vi "CUSUM_scan_histogram_20150924.vi"() -> ()   [LabVIEW 2012]
uses:
  <vilib>/Utility/file.llb/Read From Spreadsheet File (string).vi
  <vilib>/Utility/file.llb/Read From Spreadsheet File (DBL).vi
  <vilib>/Analysis/NI_AALPro.lvlib
panel:
  out "size(s)":i32[](array[numeric])=[709, 2]
  out "Bins":dbl[](array[numeric])=[0.0, 50.0, 100.0, 150.0, 200.0, 250.0, 300.0, 350.0, 400.0, 450.0, 500.0, 550.0, 600.0, 650.0, 700.0, 750.0, 800.0, 850.0, 900.0, 950.0, 1000.0, 1050.0, 1100.0, 1150.0, 1200.0, 1250.0, 1300.0, 1350.0, 1400.0, 1450.0, 1500.0, 1550.0, 1600.0, 1650.0, 1700.0, 1750.0, 1800.0, 1850.0, 1900.0, 1950.0, 2000.0, 2050.0, 2100.0, 2150.0, 2200.0, 2250.0, 2300.0, 2350.0, 2400.0, 2450.0, 2500.0, 2550.0, 2600.0, 2650.0, 2700.0, 2750.0, 2800.0, 2850.0, 2900.0, 2950.0]
  out "level histogram 2":cluster{dbl[], dbl[]}(graph)={[0.0, 50.0, 100.0, 150.0, 200.0, 250.0, 300.0, 350.0, 400.0, 450.0, 500.0, 550.0, 600.0, 650.0, 700.0, 750.0, 800.0, 850.0, 900.0, 950.0, 1000.0, 1050.0, 1100.0, 1150.0, 1200.0, 1250.0, 1300.0, 1350.0, 1400.0, 1450.0, 1500.0, 1550.0, 1600.0, 1650.0, 1700.0, 1750.0, 1800.0, 1850.0, 1900.0, 1950.0, 2000.0, 2050.0, 2100.0, 2150.0, 2200.0, 2250.0, 2300.0, 2350.0, 2400.0, 2450.0, 2500.0, 2550.0, 2600.0, 2650.0, 2700.0, 2750.0, 2800.0, 2850.0, 2900.0, 2950.0], [0.2420675662111882, 0.0, 0.0, 0.0, 0.0, 0.0024691358024691358, 0.0, 0.0, 0.0024691358024691358, 0.0011727511965947826, 0.0024691358024691358, 0.004938750687288809, 0.007694614642743324, 0.012443819440087196, 0.01625085302825151, 0.015068413748849787, 0.018650961578816, 0.022411963620084834, 0.022281722038054834, 0.014563290150013125, 0.01687631948907472, 0.029530789836521146, 0.02262728800554096, 0.02054645698593924, 0.05519131483843338, 0.02874410635546862, 0.03054171378846674, 0.01708774938009057, 0.022621934026309416, 0.014250903106779325, 0.01999323351246907, 0.02519657870780169, 0.018748477504074733, 0.011824722459045102, 0.02938347248230296, 0.03398115844900823, 0.04379840539064302, 0.05250010646123664, 0.031092530608092937, 0.020334317018267198, 0.007966809989063132, 0.01789853994964413, 0.007181120281694738, 0.007449973130269833, 0.0049692808889797374, 0.002560338394940131, 0.00022489183940309682, 0.0025128884066004968, 0.007066785952113572, 0.0, 0.0, 0.0, 0.0, 0.0024691358024691358, 0.0, 0.0, 0.0, 0.0, 0.0, 0.0]}
  out "Array 3":dbl[](array[numeric])=[98.03736431553122, 0.0, 0.0, 0.0, 0.0, 1.0, 0.0, 0.0, 1.0, 0.474964234620887, 1.0, 2.0001940283519675, 3.116318930311046, 5.039746873235314, 6.581595476441862, 6.102707568284163, 7.553639439420479, 9.076845266134358, 9.024097425412208, 5.898132510755316, 6.834909393075262, 11.959969883791064, 9.164051642244088, 8.321315079305393, 22.35248250956552, 11.641363073964792, 12.36939408432903, 6.920538498936681, 9.161883280655314, 5.771615758245627, 8.097259572549973, 10.204614376659684, 7.593133389150267, 4.789012595913266, 11.900306355332699, 13.762369171848334, 17.738354183210426, 21.26254311680084, 12.59247489627764, 8.235398392398215, 3.2265580455705685, 7.248908679605872, 2.9083537140863687, 3.0172391177592823, 2.012558760036794, 1.036937049950753, 0.09108119495825422, 1.0177198046732012, 2.8620483106059966, 0.0, 0.0, 0.0, 0.0, 1.0, 0.0, 0.0, 0.0, 0.0, 0.0, 0.0]
  out "appended array":dbl[][](array[numeric])=[[2087.0, 0.025405017525460215], [1409.93, 0.0016283498468247178], [1971.94, 0.002677117544779621], [1432.55, 0.0038086826925730686], [2003.4, 0.020381972235255154], [1492.93, 0.0007037783236276322], [2050.7, 0.0018215438964479893], [1495.13, 0.0007037783236276322], [2012.05, 0.009563105456351945], [1732.41, 0.043703253939778655], [1965.35, 0.06242927717826291], [1520.52, 0.0046642563409047], [2060.96, 0.09819777550851434], [1503.94, 0.004802252090635608], [2016.7, 0.13191013716777522], [1660.12, 0.0037672839676537962], [2047.92, 0.04607678083515028], [1878.47, 0.11755857919576077], [2132.95, 0.0061132117130792375], [1683.32, 0.05376314409516187], [2058.8, 0.11851074986890404], [1566.97, 0.0039052797173847044], [1877.93, 0.09597604393784671], [2324.51, 0.04282008114150084], [1914.27, 0.08663373168106422], [2413.94, 0.012474815775674108], [1052.8, 1.0], [956.179, 1.0], [1638.91, 0.15711947626841244], [2420.11, 0.8428805237315876], [1509.0, 1.0], [1835.61, 0.0033733701192933964], [2231.47, 0.0014518086335808613], [1816.53, 0.06200737648138094], [2191.97, 0.0007012252720226434], [1811.18, 0.004624342388557093], [2381.62, 0.0018773094054392616], [1817.39, 0.005111115271563103], [2399.92, 0.007002040701701833], [1851.14, 0.020966976034094528], [2235.07, 0.00039826872245946255], [1827.91, 0.08563458334113418], [2355.52, 0.00041018274407149776], [1847.16, 0.012768427161926872], [2282.67, 0.0007301593245090147], [1870.95, 0.0031504077148395947], [2214.97, 6.978212658477763e-05], [1794.82, 0.0021087818253302314], [2216.53, 0.00012765023155752005], [1846.39, 0.08069026437213957], [2345.59, 0.0003676326668856577], [1817.44, 0.024369280205874293], [2371.17, 0.0006212311269132643], [1824.41, 0.014817638879196926], [2385.94, 0.002399824353281377], [1990.09, 0.000719947305984413], [1585.89, 0.00012084221920778564], [1865.83, 0.0116706351705322], [2311.3, 0.000643357167049901], [1827.78, 0.01724299327878981], [2366.37, 0.003633776591670737], [1822.67, 0.014070459523813576], [2.0, 0.00013275624081982086], [1359.57, 0.012160812059713077], [710.497, 0.0006195291238258306], [1468.34, 0.07115564307633654], [1359.72, 6.808012349734402e-05], [1726.77, 0.010816229620640532], [1859.13, 0.00010382218833344963], [2062.59, 0.0012254422229521925], [1489.94, 0.0003284865958746849], [1775.88, 0.04453291078270016], [2420.58, 0.0019913436122973127], [1908.01, 0.1268264620632022], [553.398, 0.00019402835196743047], [1419.32, 0.028874482378311035], [1067.9, 0.0013207543958484742], [1319.98, 0.0012237402198647588], [1386.9, 0.0011897001581160868], [1348.68, 0.03126920072233011], [1809.94, 0.002309618189647396], [1311.37, 0.006670150099652281], [650.96, 0.0007403713430336162], [1893.96, 0.004464354098338334], [1033.78, 0.002340254245221201], [1415.39, 0.006590155954542902], [1601.36, 0.00020424037049203208], [668.442, 0.01882415414701562], [844.813, 0.0004459248089076034], [1874.38, 0.020313406848520024], [1243.4, 0.0002723204939893761], [1500.19, 0.009672483545885152], [1908.78, 0.00046464684286937297], [781.225, 0.041836937892205335], [991.016, 0.0016032869083624519], [1368.11, 0.05483683747402318], [804.302, 0.0003267845927872513], [1580.59, 0.0023147241989096966], [1227.98, 0.0006671852102739715], [1367.09, 0.018878618245813498], [1230.17, 0.0006127211114760962], [2149.49, 0.027720524285031054], [923.501, 0.00017190231183079367], [1276.66, 0.01718342317072963], [1814.61, 0.0004918788922683106], [1405.1, 0.020568707311635064], [1376.23, 0.000473156858306541], [1966.76, 0.0028406431529266795], [2346.39, 0.00041018274407149776], [1111.97, 0.010259674611049744], [891.807, 0.007575615742166956], [899.72, 1.0], [1457.06, 1.0], [1117.79, 1.0], [921.631, 1.0], [1622.73, 1.0], [1225.74, 1.0], [1085.52, 1.0], [825.602, 1.0], [1007.3, 0.017413171379768458], [1872.61, 0.9808312772822168], [1496.45, 0.0017555513380148036], [1057.57, 1.0], [1889.63, 1.0], [1572.25, 1.0], [1234.56, 1.0], [1308.71, 1.0], [877.317, 1.0], [1907.87, 1.0], [532.884, 1.0], [560.9, 1.0], [1837.08, 1.0], [737.073, 1.0], [876.931, 1.0], [1432.36, 1.0], [993.583, 1.0], [1912.61, 1.0], [1794.02, 1.0], [1006.65, 1.0], [1036.25, 0.53125], [1896.78, 0.46875], [1241.31, 1.0], [267.724, 1.0], [1864.09, 1.0], [1112.04, 1.0], [1715.8, 1.0], [1014.02, 1.0], [1930.18, 1.0], [1560.29, 1.0], [656.028, 1.0], [682.156, 1.0], [912.345, 1.0], [1527.18, 1.0], [1627.9, 1.0], [1981.19, 0.0986159169550173], [1304.79, 0.23269896193771628], [719.808, 0.6686851211072664], [1456.22, 1.0], [1415.17, 1.0], [1870.44, 1.0], [1203.85, 1.0], [1745.38, 1.0], [1213.0, 1.0], [1933.99, 1.0], [1377.11, 1.0], [2071.24, 1.0], [1299.64, 1.0], [1606.14, 1.0], [1333.08, 1.0], [1854.4, 1.0], [1301.7, 0.17391304347826086], [1945.79, 0.8260869565217391], [1563.82, 1.0], [1910.86, 1.0], [1317.53, 1.0], [1695.63, 0.9234449760765551], [1301.8, 0.07655502392344497], [1869.95, 1.0], [1242.76, 1.0], [1788.06, 1.0], [1218.82, 1.0], [1804.39, 1.0], [1221.43, 1.0], [1810.53, 1.0], [1234.33, 1.0], [1555.4, 0.8295454545454546], [1255.86, 0.17045454545454544], [1631.74, 1.0], [1219.12, 1.0], [1684.0, 1.0], [1323.78, 0.2111111111111111], [1442.83, 0.7888888888888889], [1434.86, 1.0], [893.039, 1.0], [1474.1, 0.21739130434782608], [1657.34, 0.782608695652174], [2172.57, 1.0], [1728.16, 1.0], [2227.86, 1.0], [697.854, 1.0], [1157.3, 1.0], [851.024, 1.0], [2082.22, 1.0], [1218.51, 1.0], [1243.71, 1.0], [2094.94, 1.0], [1419.8, 0.015584415584415584], [2150.5, 0.007956600361663653], [1398.3, 0.006444188722669736], [1553.93, 0.010126582278481013], [1349.85, 0.003616636528028933], [825.641, 0.003222094361334868], [1322.58, 0.0564852868650337], [2175.33, 0.008581292125595923], [1316.6, 0.0017425612362321223], [1665.94, 0.009436133486766397], [1191.15, 0.008022357389445997], [1846.44, 0.002564524083511425], [808.1, 0.038895281933256615], [1868.78, 0.0015124116389939174], [1512.96, 0.01594607923721848], [1786.59, 0.0018083182640144665], [2325.2, 0.02857142857142857], [1783.95, 0.02314647377938517], [2290.33, 0.018411967779056387], [1778.8, 0.003090580305770179], [1461.36, 0.0010192339306263358], [1776.12, 0.00404405720861417], [1383.75, 0.022258753904323525], [2046.5, 0.003748150583593622], [1726.44, 0.00805523590333717], [2060.53, 0.003748150583593622], [1778.36, 0.0015124116389939174], [2039.58, 0.026631596251849417], [1766.09, 0.016570771001150748], [2416.11, 0.004701627486437613], [1796.06, 0.010290974847936873], [2358.84, 0.0017754397501232944], [1872.71, 0.001906953805687983], [695.836, 0.0018083182640144665], [1652.45, 0.010488245931283906], [1904.68, 0.027946736807496302], [1506.86, 0.026927502876869965], [1966.76, 0.0007562058194969587], [1978.89, 0.03524576689133651], [1397.85, 0.0012493835278645405], [1876.81, 0.003846786125267138], [940.985, 0.00496465559756699], [1864.98, 0.012230807167516029], [826.127, 0.003024823277987835], [1709.33, 0.011507479861910242], [1087.22, 0.03665954298865691], [1665.07, 0.0014795331251027453], [1506.68, 0.010685517014630939], [1800.97, 0.01818181818181818], [616.846, 0.03307578497451915], [1702.82, 0.029360512904816703], [793.399, 0.015091237876048002], [884.288, 0.016340621403912542], [810.608, 0.007266151569949039], [1895.02, 0.035771823113595266], [801.773, 0.03471971066907776], [625.159, 0.010323853361828046], [1425.1, 0.0020384678612526716], [1741.45, 0.012855498931448299], [1267.96, 0.003813907611375966], [1358.47, 0.06625020549071182], [1036.84, 0.029360512904816703], [1216.22, 0.002498767055729081], [1095.59, 0.0020055893473614993], [1612.34, 0.011704750945257275], [1690.86, 0.0020713463751438435], [645.438, 0.035147131349663], [1878.73, 0.0102580963340457], [1371.09, 0.019069538056879828], [1845.36, 0.0021042248890350158], [1213.25, 0.02975505507151077], [1477.36, 0.010685517014630939], [2093.92, 1.0], [1182.64, 1.0], [985.497, 1.0], [1612.24, 1.0], [1447.08, 1.0], [890.263, 0.01613181009242781], [722.736, 0.5019231873241863], [1935.48, 0.020265227625007175], [834.119, 0.4616797749583788], [1995.94, 1.0], [1864.17, 1.0], [1166.73, 1.0], [1955.6, 1.0], [1806.84, 1.0], [1864.15, 0.05513784461152882], [1920.31, 0.9448621553884712], [1545.9, 1.0], [1982.65, 1.0], [1836.01, 1.0], [1357.88, 1.0], [1120.61, 1.0], [1730.66, 1.0], [965.86, 0.19097395055583208], [1072.11, 0.004604280736684918], [1322.99, 0.7866268458602953], [2255.49, 0.017794922847187655], [1444.9, 1.0], [1965.5, 1.0], [644.821, 1.0], [1108.12, 1.0], [1302.96, 1.0], [1899.61, 0.0031546159893585616], [1454.0, 0.0010150499397936065], [967.774, 0.03946421285530894], [1500.54, 0.0020201484095892365], [896.694, 0.036661215472545555], [1901.57, 0.00021561518328949158], [1594.48, 0.06215024729402945], [847.541, 0.0012439337497470667], [1809.79, 0.013195649217316885], [934.503, 0.018960867502811292], [872.881, 0.0001360034233056793], [2120.85, 0.7135502532649114], [1227.66, 0.0009188523964798334], [1891.14, 0.06534466916337991], [1098.81, 0.0012704710030750042], [780.638, 0.03454818667630854], [691.653, 0.006150008458749499], [1426.0, 1.0], [553.58, 1.0], [1783.21, 0.5357142857142857], [1219.72, 0.4642857142857143], [1707.02, 0.16176470588235295], [1217.79, 0.8382352941176471], [1805.49, 1.0], [1217.83, 1.0], [1760.29, 1.0], [1215.47, 1.0], [1661.88, 1.0], [1370.49, 1.0], [1709.93, 1.0], [1216.34, 1.0], [2388.41, 1.0], [1836.91, 1.0], [2110.84, 1.0], [1895.06, 1.0], [2403.14, 1.0], [1741.31, 1.0], [1217.33, 1.0], [1784.55, 1.0], [1229.73, 1.0], [1862.39, 1.0], [806.501, 1.0], [731.362, 0.3125], [1873.14, 0.6875], [906.667, 1.0], [1082.78, 1.0], [1886.99, 1.0], [1228.77, 1.0], [1944.18, 1.0], [1885.95, 1.0], [1574.2, 1.0], [782.094, 1.0], [846.688, 1.0], [1020.4, 1.0], [965.63, 1.0], [1532.01, 1.0], [1577.86, 1.0], [2070.04, 1.0], [1292.32, 1.0], [1585.95, 1.0], [727.528, 1.0], [925.014, 1.0], [414.909, 1.0], [927.775, 1.0], [1106.07, 1.0], [2188.58, 1.0], [1868.95, 1.0], [1725.62, 1.0], [1064.71, 1.0], [813.617, 1.0], [801.414, 1.0], [797.952, 1.0], [1464.53, 0.4668574153552694], [1848.46, 0.058178350023843584], [479.276, 0.474964234620887], [717.31, 1.0], [1851.48, 1.0], [1715.99, 1.0], [1203.69, 1.0], [1200.54, 1.0], [1485.82, 1.0], [1892.21, 0.1884328358208955], [1337.15, 0.19029850746268656], [1824.55, 0.31529850746268656], [1302.31, 0.2891791044776119], [1802.99, 0.016791044776119403], [1270.27, 1.0], [1842.57, 1.0], [1282.09, 1.0], [1591.09, 1.0], [1798.15, 1.0], [1955.94, 1.0], [1282.86, 1.0], [1928.13, 1.0], [1326.64, 1.0], [1836.94, 1.0], [1235.91, 1.0], [1801.4, 1.0], [1273.72, 1.0], [1814.73, 1.0], [1302.86, 0.09285714285714286], [1825.97, 0.9071428571428571], [1463.64, 1.0], [1957.29, 1.0], [1290.55, 1.0], [1830.68, 1.0], [1345.13, 1.0], [1976.41, 1.0], [1344.34, 0.2121020154383989], [1730.56, 0.0012083245348537106], [1939.82, 0.17236808146219], [772.718, 0.0029445578470706927], [1148.21, 0.03011426292203374], [2232.36, 0.010511250322610919], [1905.87, 0.03345768517866779], [1203.01, 0.005642758264705192], [1800.68, 0.0004340583280542456], [664.521, 0.012224021022500645], [1141.53, 0.014112761314844794], [1423.25, 0.11152952769761386], [977.888, 0.06548415100537294], [1285.93, 0.0019473968231622908], [710.905, 0.05070270523920133], [1897.52, 0.04152882381924403], [1632.4, 0.01031181811782924], [1876.66, 0.1625724408155604], [1181.2, 0.0052321625489782034], [1863.87, 0.05429248492527158], [1187.18, 0.0012787123718354801], [763.809, 1.0], [1523.82, 1.0], [1034.17, 1.0], [1308.35, 1.0], [1296.01, 0.29411764705882354], [1352.97, 0.7058823529411765], [1594.5, 0.23636363636363636], [1926.88, 0.7636363636363637], [800.235, 1.0], [1014.41, 1.0], [1319.65, 1.0], [2084.98, 1.0], [1738.27, 1.0], [1066.1, 1.0], [923.378, 1.0], [2678.15, 1.0], [1368.67, 1.0], [1126.06, 1.0], [1298.0, 1.0], [2226.06, 1.0], [1084.34, 1.0], [1197.12, 1.0], [2082.17, 1.0], [1084.2, 1.0], [1825.56, 1.0], [1767.73, 1.0], [628.111, 1.0], [1847.57, 1.0], [1757.86, 1.0], [1137.1, 1.0], [1015.28, 1.0], [1879.5, 0.15833333333333333], [1720.65, 0.8416666666666667], [1251.11, 1.0], [1893.86, 1.0], [668.096, 1.0], [1779.05, 1.0], [872.978, 1.0], [1874.4, 0.004883093008559775], [1574.83, 0.02892514505658643], [1836.68, 0.009220428563221693], [1656.86, 0.00195323720342391], [2122.34, 0.15427701499396795], [1837.76, 0.0029585798816568047], [1183.61, 0.047768139254322974], [705.432, 0.002297926121675188], [639.157, 0.037772160625035904], [1874.69, 0.003159648417303384], [1176.06, 0.007066122824151203], [1401.87, 0.0642270351008215], [1375.3, 0.006204400528523008], [1807.7, 0.0053714023094157525], [1284.45, 0.1105589705290975], [1730.3, 0.010513012006663986], [1243.8, 0.004883093008559775], [1887.93, 0.006290572758085828], [1289.93, 0.04328718331705635], [1753.03, 0.0023840983512380077], [1419.85, 0.07494111564313208], [2019.86, 0.005342678232894813], [1753.86, 0.0046820244729131955], [1407.8, 0.026426150399264662], [1539.38, 0.002700063192968346], [2007.24, 0.0030734761877405643], [1163.74, 0.02260584822197966], [1946.82, 0.003504337335554662], [1965.55, 0.03211351755041075], [702.695, 0.0045096800137875565], [1701.36, 0.0055437467685413916], [1379.27, 0.0013213075199632331], [1787.09, 0.04748089848911358], [1341.8, 0.003044752111219624], [1235.84, 0.004710748549434136], [1103.74, 0.003504337335554662], [1839.3, 0.059401390245303616], [747.021, 0.006233124605043948], [743.118, 0.034124202906876545], [1797.89, 0.007238467283276842], [1793.13, 0.041132877577985866], [1426.95, 0.003705405871201241], [2125.28, 0.0066927098293789854], [1782.71, 0.016631240305624174], [2302.87, 0.018268512667317747], [846.165, 0.0028149594990521053], [1397.34, 0.004251163325099098], [756.643, 1.0], [1183.51, 1.0], [786.257, 1.0], [781.436, 1.0], [690.436, 1.0], [1085.61, 1.0], [1480.42, 1.0], [1772.17, 1.0], [1768.87, 1.0], [1128.08, 1.0], [1780.1, 1.0], [1585.3, 1.0], [1270.53, 1.0], [906.421, 1.0], [1911.6, 1.0], [1357.53, 1.0], [1840.69, 1.0], [836.077, 1.0], [1310.64, 1.0], [1881.75, 1.0], [2187.62, 1.0], [1534.2, 1.0], [1152.6, 1.0], [965.228, 1.0], [907.996, 1.0], [1049.23, 0.2545454545454545], [1711.8, 0.7454545454545455], [2030.86, 1.0], [1853.24, 1.0], [1064.62, 0.020169851380042462], [2026.48, 0.9798301486199575], [1169.14, 1.0], [2425.73, 1.0], [2266.82, 1.0], [893.285, 1.0], [1299.6, 1.0], [1615.69, 1.0], [1955.45, 1.0], [1084.31, 1.0], [1546.11, 1.0], [1529.82, 1.0], [1816.24, 1.0], [2148.28, 1.0], [1410.36, 1.0], [1552.85, 1.0], [1781.22, 1.0], [1780.3, 1.0], [1697.19, 1.0], [1190.53, 1.0], [1069.78, 0.8939393939393939], [1108.17, 0.10606060606060606], [1851.27, 1.0], [1342.98, 1.0], [850.381, 1.0], [1854.66, 1.0], [1398.03, 1.0], [1100.29, 1.0], [2016.17, 1.0], [1625.97, 0.41379310344827586], [1941.51, 0.5862068965517241], [701.989, 1.0], [1930.6, 1.0], [1708.51, 1.0], [942.204, 1.0], [1067.87, 1.0], [709.937, 1.0], [1600.57, 1.0], [1412.42, 1.0], [648.139, 1.0], [1877.51, 1.0], [885.259, 1.0], [954.4, 0.03443043884220355], [997.229, 0.39017273576097106], [1723.12, 0.017857142857142856], [1855.66, 0.042600373482726425], [974.682, 0.035130718954248366], [1400.0, 0.013071895424836602], [753.804, 0.008286647992530346], [1554.74, 0.031162464985994398], [986.868, 0.14087301587301587], [1524.19, 0.01984126984126984], [1155.7, 0.22934173669467786], [0.0, 0.03723155929038282], [0.0, 0.07675438596491228], [0.0, 0.9232456140350878], [0.0, 1.0], [0.0, 1.0], [0.0, 1.0], [0.0, 1.0], [0.0, 1.0], [0.0, 1.0], [0.0, 1.0], [0.0, 1.0], [0.0, 1.0], [0.0, 1.0], [0.0, 1.0], [0.0, 1.0], [0.0, 1.0], [0.0, 1.0], [0.0, 1.0], [0.0, 1.0], [0.0, 1.0], [0.0, 1.0], [0.0, 1.0], [0.0, 1.0], [0.0, 1.0], [0.0, 1.0], [0.0, 1.0], [0.0, 1.0], [0.0, 1.0], [0.0, 1.0], [0.0, 1.0], [0.0, 1.0], [0.0, 1.0], [0.0, 1.0], [0.0, 1.0], [0.0, 1.0], [0.0, 1.0], [0.0, 1.0], [0.0, 1.0], [0.0, 1.0], [0.0, 1.0], [0.0, 0.03875], [0.0, 0.87125], [0.0, 0.09], [0.0, 1.0], [0.0, 1.0], [0.0, 1.0], [0.0, 1.0], [0.0, 1.0], [0.0, 0.2927170868347339], [0.0, 0.7072829131652661], [0.0, 1.0], [0.0, 1.0], [0.0, 1.0], [0.0, 1.0], [0.0, 1.0], [0.0, 1.0], [0.0, 1.0], [0.0, 1.0], [0.0, 1.0], [0.0, 1.0], [0.0, 1.0], [0.0, 1.0], [0.0, 1.0], [0.0, 0.46153846153846156], [0.0, 0.5384615384615384], [0.0, 1.0], [0.0, 1.0], [0.0, 1.0], [0.0, 1.0], [0.0, 1.0], [0.0, 1.0], [0.0, 1.0], [0.0, 1.0], [0.0, 1.0], [0.0, 1.0], [0.0, 1.0], [0.0, 1.0], [0.0, 1.0], [0.0, 1.0], [0.0, 1.0], [0.0, 1.0], [0.0, 1.0], [0.0, 1.0], [0.0, 1.0], [0.0, 1.0], [0.0, 1.0], [0.0, 1.0], [0.0, 1.0], [0.0, 1.0], [0.0, 1.0], [0.0, 1.0], [0.0, 1.0], [0.0, 1.0], [0.0, 1.0], [0.0, 1.0], [0.0, 1.0], [0.0, 1.0], [0.0, 1.0], [0.0, 1.0], [0.0, 1.0], [0.0, 1.0], [0.0, 1.0], [0.0, 1.0], [0.0, 1.0]]
  out "Array 2":dbl[](array[numeric])=[0.025405017525460215, 0.0016283498468247178, 0.002677117544779621, 0.0038086826925730686, 0.020381972235255154, 0.0007037783236276322, 0.0018215438964479893, 0.0007037783236276322, 0.009563105456351945, 0.043703253939778655, 0.06242927717826291, 0.0046642563409047, 0.09819777550851434, 0.004802252090635608, 0.13191013716777522, 0.0037672839676537962, 0.04607678083515028, 0.11755857919576077, 0.0061132117130792375, 0.05376314409516187, 0.11851074986890404, 0.0039052797173847044, 0.09597604393784671, 0.04282008114150084, 0.08663373168106422, 0.012474815775674108, 1.0, 1.0, 0.15711947626841244, 0.8428805237315876, 1.0, 0.0033733701192933964, 0.0014518086335808613, 0.06200737648138094, 0.0007012252720226434, 0.004624342388557093, 0.0018773094054392616, 0.005111115271563103, 0.007002040701701833, 0.020966976034094528, 0.00039826872245946255, 0.08563458334113418, 0.00041018274407149776, 0.012768427161926872, 0.0007301593245090147, 0.0031504077148395947, 6.978212658477763e-05, 0.0021087818253302314, 0.00012765023155752005, 0.08069026437213957, 0.0003676326668856577, 0.024369280205874293, 0.0006212311269132643, 0.014817638879196926, 0.002399824353281377, 0.000719947305984413, 0.00012084221920778564, 0.0116706351705322, 0.000643357167049901, 0.01724299327878981, 0.003633776591670737, 0.014070459523813576, 0.00013275624081982086, 0.012160812059713077, 0.0006195291238258306, 0.07115564307633654, 6.808012349734402e-05, 0.010816229620640532, 0.00010382218833344963, 0.0012254422229521925, 0.0003284865958746849, 0.04453291078270016, 0.0019913436122973127, 0.1268264620632022, 0.00019402835196743047, 0.028874482378311035, 0.0013207543958484742, 0.0012237402198647588, 0.0011897001581160868, 0.03126920072233011, 0.002309618189647396, 0.006670150099652281, 0.0007403713430336162, 0.004464354098338334, 0.002340254245221201, 0.006590155954542902, 0.00020424037049203208, 0.01882415414701562, 0.0004459248089076034, 0.020313406848520024, 0.0002723204939893761, 0.009672483545885152, 0.00046464684286937297, 0.041836937892205335, 0.0016032869083624519, 0.05483683747402318, 0.0003267845927872513, 0.0023147241989096966, 0.0006671852102739715, 0.018878618245813498, 0.0006127211114760962, 0.027720524285031054, 0.00017190231183079367, 0.01718342317072963, 0.0004918788922683106, 0.020568707311635064, 0.000473156858306541, 0.0028406431529266795, 0.00041018274407149776, 0.010259674611049744, 0.007575615742166956, 1.0, 1.0, 1.0, 1.0, 1.0, 1.0, 1.0, 1.0, 0.017413171379768458, 0.9808312772822168, 0.0017555513380148036, 1.0, 1.0, 1.0, 1.0, 1.0, 1.0, 1.0, 1.0, 1.0, 1.0, 1.0, 1.0, 1.0, 1.0, 1.0, 1.0, 1.0, 0.53125, 0.46875, 1.0, 1.0, 1.0, 1.0, 1.0, 1.0, 1.0, 1.0, 1.0, 1.0, 1.0, 1.0, 1.0, 0.0986159169550173, 0.23269896193771628, 0.6686851211072664, 1.0, 1.0, 1.0, 1.0, 1.0, 1.0, 1.0, 1.0, 1.0, 1.0, 1.0, 1.0, 1.0, 0.17391304347826086, 0.8260869565217391, 1.0, 1.0, 1.0, 0.9234449760765551, 0.07655502392344497, 1.0, 1.0, 1.0, 1.0, 1.0, 1.0, 1.0, 1.0, 0.8295454545454546, 0.17045454545454544, 1.0, 1.0, 1.0, 0.2111111111111111, 0.7888888888888889, 1.0, 1.0, 0.21739130434782608, 0.782608695652174, 1.0, 1.0, 1.0, 1.0, 1.0, 1.0, 1.0, 1.0, 1.0, 1.0, 0.015584415584415584, 0.007956600361663653, 0.006444188722669736, 0.010126582278481013, 0.003616636528028933, 0.003222094361334868, 0.0564852868650337, 0.008581292125595923, 0.0017425612362321223, 0.009436133486766397, 0.008022357389445997, 0.002564524083511425, 0.038895281933256615, 0.0015124116389939174, 0.01594607923721848, 0.0018083182640144665, 0.02857142857142857, 0.02314647377938517, 0.018411967779056387, 0.003090580305770179, 0.0010192339306263358, 0.00404405720861417, 0.022258753904323525, 0.003748150583593622, 0.00805523590333717, 0.003748150583593622, 0.0015124116389939174, 0.026631596251849417, 0.016570771001150748, 0.004701627486437613, 0.010290974847936873, 0.0017754397501232944, 0.001906953805687983, 0.0018083182640144665, 0.010488245931283906, 0.027946736807496302, 0.026927502876869965, 0.0007562058194969587, 0.03524576689133651, 0.0012493835278645405, 0.003846786125267138, 0.00496465559756699, 0.012230807167516029, 0.003024823277987835, 0.011507479861910242, 0.03665954298865691, 0.0014795331251027453, 0.010685517014630939, 0.01818181818181818, 0.03307578497451915, 0.029360512904816703, 0.015091237876048002, 0.016340621403912542, 0.007266151569949039, 0.035771823113595266, 0.03471971066907776, 0.010323853361828046, 0.0020384678612526716, 0.012855498931448299, 0.003813907611375966, 0.06625020549071182, 0.029360512904816703, 0.002498767055729081, 0.0020055893473614993, 0.011704750945257275, 0.0020713463751438435, 0.035147131349663, 0.0102580963340457, 0.019069538056879828, 0.0021042248890350158, 0.02975505507151077, 0.010685517014630939, 1.0, 1.0, 1.0, 1.0, 1.0, 0.01613181009242781, 0.5019231873241863, 0.020265227625007175, 0.4616797749583788, 1.0, 1.0, 1.0, 1.0, 1.0, 0.05513784461152882, 0.9448621553884712, 1.0, 1.0, 1.0, 1.0, 1.0, 1.0, 0.19097395055583208, 0.004604280736684918, 0.7866268458602953, 0.017794922847187655, 1.0, 1.0, 1.0, 1.0, 1.0, 0.0031546159893585616, 0.0010150499397936065, 0.03946421285530894, 0.0020201484095892365, 0.036661215472545555, 0.00021561518328949158, 0.06215024729402945, 0.0012439337497470667, 0.013195649217316885, 0.018960867502811292, 0.0001360034233056793, 0.7135502532649114, 0.0009188523964798334, 0.06534466916337991, 0.0012704710030750042, 0.03454818667630854, 0.006150008458749499, 1.0, 1.0, 0.5357142857142857, 0.4642857142857143, 0.16176470588235295, 0.8382352941176471, 1.0, 1.0, 1.0, 1.0, 1.0, 1.0, 1.0, 1.0, 1.0, 1.0, 1.0, 1.0, 1.0, 1.0, 1.0, 1.0, 1.0, 1.0, 1.0, 0.3125, 0.6875, 1.0, 1.0, 1.0, 1.0, 1.0, 1.0, 1.0, 1.0, 1.0, 1.0, 1.0, 1.0, 1.0, 1.0, 1.0, 1.0, 1.0, 1.0, 1.0, 1.0, 1.0, 1.0, 1.0, 1.0, 1.0, 1.0, 1.0, 1.0, 0.4668574153552694, 0.058178350023843584, 0.474964234620887, 1.0, 1.0, 1.0, 1.0, 1.0, 1.0, 0.1884328358208955, 0.19029850746268656, 0.31529850746268656, 0.2891791044776119, 0.016791044776119403, 1.0, 1.0, 1.0, 1.0, 1.0, 1.0, 1.0, 1.0, 1.0, 1.0, 1.0, 1.0, 1.0, 1.0, 0.09285714285714286, 0.9071428571428571, 1.0, 1.0, 1.0, 1.0, 1.0, 1.0, 0.2121020154383989, 0.0012083245348537106, 0.17236808146219, 0.0029445578470706927, 0.03011426292203374, 0.010511250322610919, 0.03345768517866779, 0.005642758264705192, 0.0004340583280542456, 0.012224021022500645, 0.014112761314844794, 0.11152952769761386, 0.06548415100537294, 0.0019473968231622908, 0.05070270523920133, 0.04152882381924403, 0.01031181811782924, 0.1625724408155604, 0.0052321625489782034, 0.05429248492527158, 0.0012787123718354801, 1.0, 1.0, 1.0, 1.0, 0.29411764705882354, 0.7058823529411765, 0.23636363636363636, 0.7636363636363637, 1.0, 1.0, 1.0, 1.0, 1.0, 1.0, 1.0, 1.0, 1.0, 1.0, 1.0, 1.0, 1.0, 1.0, 1.0, 1.0, 1.0, 1.0, 1.0, 1.0, 1.0, 1.0, 1.0, 0.15833333333333333, 0.8416666666666667, 1.0, 1.0, 1.0, 1.0, 1.0, 0.004883093008559775, 0.02892514505658643, 0.009220428563221693, 0.00195323720342391, 0.15427701499396795, 0.0029585798816568047, 0.047768139254322974, 0.002297926121675188, 0.037772160625035904, 0.003159648417303384, 0.007066122824151203, 0.0642270351008215, 0.006204400528523008, 0.0053714023094157525, 0.1105589705290975, 0.010513012006663986, 0.004883093008559775, 0.006290572758085828, 0.04328718331705635, 0.0023840983512380077, 0.07494111564313208, 0.005342678232894813, 0.0046820244729131955, 0.026426150399264662, 0.002700063192968346, 0.0030734761877405643, 0.02260584822197966, 0.003504337335554662, 0.03211351755041075, 0.0045096800137875565, 0.0055437467685413916, 0.0013213075199632331, 0.04748089848911358, 0.003044752111219624, 0.004710748549434136, 0.003504337335554662, 0.059401390245303616, 0.006233124605043948, 0.034124202906876545, 0.007238467283276842, 0.041132877577985866, 0.003705405871201241, 0.0066927098293789854, 0.016631240305624174, 0.018268512667317747, 0.0028149594990521053, 0.004251163325099098, 1.0, 1.0, 1.0, 1.0, 1.0, 1.0, 1.0, 1.0, 1.0, 1.0, 1.0, 1.0, 1.0, 1.0, 1.0, 1.0, 1.0, 1.0, 1.0, 1.0, 1.0, 1.0, 1.0, 1.0, 1.0, 0.2545454545454545, 0.7454545454545455, 1.0, 1.0, 0.020169851380042462, 0.9798301486199575, 1.0, 1.0, 1.0, 1.0, 1.0, 1.0, 1.0, 1.0, 1.0, 1.0, 1.0, 1.0, 1.0, 1.0, 1.0, 1.0, 1.0, 1.0, 0.8939393939393939, 0.10606060606060606, 1.0, 1.0, 1.0, 1.0, 1.0, 1.0, 1.0, 0.41379310344827586, 0.5862068965517241, 1.0, 1.0, 1.0, 1.0, 1.0, 1.0, 1.0, 1.0, 1.0, 1.0, 1.0, 0.03443043884220355, 0.39017273576097106, 0.017857142857142856, 0.042600373482726425, 0.035130718954248366, 0.013071895424836602, 0.008286647992530346, 0.031162464985994398, 0.14087301587301587, 0.01984126984126984, 0.22934173669467786, 0.03723155929038282, 0.07675438596491228, 0.9232456140350878, 1.0, 1.0, 1.0, 1.0, 1.0, 1.0, 1.0, 1.0, 1.0, 1.0, 1.0, 1.0, 1.0, 1.0, 1.0, 1.0, 1.0, 1.0, 1.0, 1.0, 1.0, 1.0, 1.0, 1.0, 1.0, 1.0, 1.0, 1.0, 1.0, 1.0, 1.0, 1.0, 1.0, 1.0, 1.0, 1.0, 1.0, 0.03875, 0.87125, 0.09, 1.0, 1.0, 1.0, 1.0, 1.0, 0.2927170868347339, 0.7072829131652661, 1.0, 1.0, 1.0, 1.0, 1.0, 1.0, 1.0, 1.0, 1.0, 1.0, 1.0, 1.0, 1.0, 0.46153846153846156, 0.5384615384615384, 1.0, 1.0, 1.0, 1.0, 1.0, 1.0, 1.0, 1.0, 1.0, 1.0, 1.0, 1.0, 1.0, 1.0, 1.0, 1.0, 1.0, 1.0, 1.0, 1.0, 1.0, 1.0, 1.0, 1.0, 1.0, 1.0, 1.0, 1.0, 1.0, 1.0, 1.0, 1.0, 1.0, 1.0, 1.0, 1.0, 1.0, 1.0, 1.0]
  out "Array":dbl[](array[numeric])=[2087.0, 1409.93, 1971.94, 1432.55, 2003.4, 1492.93, 2050.7, 1495.13, 2012.05, 1732.41, 1965.35, 1520.52, 2060.96, 1503.94, 2016.7, 1660.12, 2047.92, 1878.47, 2132.95, 1683.32, 2058.8, 1566.97, 1877.93, 2324.51, 1914.27, 2413.94, 1052.8, 956.179, 1638.91, 2420.11, 1509.0, 1835.61, 2231.47, 1816.53, 2191.97, 1811.18, 2381.62, 1817.39, 2399.92, 1851.14, 2235.07, 1827.91, 2355.52, 1847.16, 2282.67, 1870.95, 2214.97, 1794.82, 2216.53, 1846.39, 2345.59, 1817.44, 2371.17, 1824.41, 2385.94, 1990.09, 1585.89, 1865.83, 2311.3, 1827.78, 2366.37, 1822.67, 2.0, 1359.57, 710.497, 1468.34, 1359.72, 1726.77, 1859.13, 2062.59, 1489.94, 1775.88, 2420.58, 1908.01, 553.398, 1419.32, 1067.9, 1319.98, 1386.9, 1348.68, 1809.94, 1311.37, 650.96, 1893.96, 1033.78, 1415.39, 1601.36, 668.442, 844.813, 1874.38, 1243.4, 1500.19, 1908.78, 781.225, 991.016, 1368.11, 804.302, 1580.59, 1227.98, 1367.09, 1230.17, 2149.49, 923.501, 1276.66, 1814.61, 1405.1, 1376.23, 1966.76, 2346.39, 1111.97, 891.807, 899.72, 1457.06, 1117.79, 921.631, 1622.73, 1225.74, 1085.52, 825.602, 1007.3, 1872.61, 1496.45, 1057.57, 1889.63, 1572.25, 1234.56, 1308.71, 877.317, 1907.87, 532.884, 560.9, 1837.08, 737.073, 876.931, 1432.36, 993.583, 1912.61, 1794.02, 1006.65, 1036.25, 1896.78, 1241.31, 267.724, 1864.09, 1112.04, 1715.8, 1014.02, 1930.18, 1560.29, 656.028, 682.156, 912.345, 1527.18, 1627.9, 1981.19, 1304.79, 719.808, 1456.22, 1415.17, 1870.44, 1203.85, 1745.38, 1213.0, 1933.99, 1377.11, 2071.24, 1299.64, 1606.14, 1333.08, 1854.4, 1301.7, 1945.79, 1563.82, 1910.86, 1317.53, 1695.63, 1301.8, 1869.95, 1242.76, 1788.06, 1218.82, 1804.39, 1221.43, 1810.53, 1234.33, 1555.4, 1255.86, 1631.74, 1219.12, 1684.0, 1323.78, 1442.83, 1434.86, 893.039, 1474.1, 1657.34, 2172.57, 1728.16, 2227.86, 697.854, 1157.3, 851.024, 2082.22, 1218.51, 1243.71, 2094.94, 1419.8, 2150.5, 1398.3, 1553.93, 1349.85, 825.641, 1322.58, 2175.33, 1316.6, 1665.94, 1191.15, 1846.44, 808.1, 1868.78, 1512.96, 1786.59, 2325.2, 1783.95, 2290.33, 1778.8, 1461.36, 1776.12, 1383.75, 2046.5, 1726.44, 2060.53, 1778.36, 2039.58, 1766.09, 2416.11, 1796.06, 2358.84, 1872.71, 695.836, 1652.45, 1904.68, 1506.86, 1966.76, 1978.89, 1397.85, 1876.81, 940.985, 1864.98, 826.127, 1709.33, 1087.22, 1665.07, 1506.68, 1800.97, 616.846, 1702.82, 793.399, 884.288, 810.608, 1895.02, 801.773, 625.159, 1425.1, 1741.45, 1267.96, 1358.47, 1036.84, 1216.22, 1095.59, 1612.34, 1690.86, 645.438, 1878.73, 1371.09, 1845.36, 1213.25, 1477.36, 2093.92, 1182.64, 985.497, 1612.24, 1447.08, 890.263, 722.736, 1935.48, 834.119, 1995.94, 1864.17, 1166.73, 1955.6, 1806.84, 1864.15, 1920.31, 1545.9, 1982.65, 1836.01, 1357.88, 1120.61, 1730.66, 965.86, 1072.11, 1322.99, 2255.49, 1444.9, 1965.5, 644.821, 1108.12, 1302.96, 1899.61, 1454.0, 967.774, 1500.54, 896.694, 1901.57, 1594.48, 847.541, 1809.79, 934.503, 872.881, 2120.85, 1227.66, 1891.14, 1098.81, 780.638, 691.653, 1426.0, 553.58, 1783.21, 1219.72, 1707.02, 1217.79, 1805.49, 1217.83, 1760.29, 1215.47, 1661.88, 1370.49, 1709.93, 1216.34, 2388.41, 1836.91, 2110.84, 1895.06, 2403.14, 1741.31, 1217.33, 1784.55, 1229.73, 1862.39, 806.501, 731.362, 1873.14, 906.667, 1082.78, 1886.99, 1228.77, 1944.18, 1885.95, 1574.2, 782.094, 846.688, 1020.4, 965.63, 1532.01, 1577.86, 2070.04, 1292.32, 1585.95, 727.528, 925.014, 414.909, 927.775, 1106.07, 2188.58, 1868.95, 1725.62, 1064.71, 813.617, 801.414, 797.952, 1464.53, 1848.46, 479.276, 717.31, 1851.48, 1715.99, 1203.69, 1200.54, 1485.82, 1892.21, 1337.15, 1824.55, 1302.31, 1802.99, 1270.27, 1842.57, 1282.09, 1591.09, 1798.15, 1955.94, 1282.86, 1928.13, 1326.64, 1836.94, 1235.91, 1801.4, 1273.72, 1814.73, 1302.86, 1825.97, 1463.64, 1957.29, 1290.55, 1830.68, 1345.13, 1976.41, 1344.34, 1730.56, 1939.82, 772.718, 1148.21, 2232.36, 1905.87, 1203.01, 1800.68, 664.521, 1141.53, 1423.25, 977.888, 1285.93, 710.905, 1897.52, 1632.4, 1876.66, 1181.2, 1863.87, 1187.18, 763.809, 1523.82, 1034.17, 1308.35, 1296.01, 1352.97, 1594.5, 1926.88, 800.235, 1014.41, 1319.65, 2084.98, 1738.27, 1066.1, 923.378, 2678.15, 1368.67, 1126.06, 1298.0, 2226.06, 1084.34, 1197.12, 2082.17, 1084.2, 1825.56, 1767.73, 628.111, 1847.57, 1757.86, 1137.1, 1015.28, 1879.5, 1720.65, 1251.11, 1893.86, 668.096, 1779.05, 872.978, 1874.4, 1574.83, 1836.68, 1656.86, 2122.34, 1837.76, 1183.61, 705.432, 639.157, 1874.69, 1176.06, 1401.87, 1375.3, 1807.7, 1284.45, 1730.3, 1243.8, 1887.93, 1289.93, 1753.03, 1419.85, 2019.86, 1753.86, 1407.8, 1539.38, 2007.24, 1163.74, 1946.82, 1965.55, 702.695, 1701.36, 1379.27, 1787.09, 1341.8, 1235.84, 1103.74, 1839.3, 747.021, 743.118, 1797.89, 1793.13, 1426.95, 2125.28, 1782.71, 2302.87, 846.165, 1397.34, 756.643, 1183.51, 786.257, 781.436, 690.436, 1085.61, 1480.42, 1772.17, 1768.87, 1128.08, 1780.1, 1585.3, 1270.53, 906.421, 1911.6, 1357.53, 1840.69, 836.077, 1310.64, 1881.75, 2187.62, 1534.2, 1152.6, 965.228, 907.996, 1049.23, 1711.8, 2030.86, 1853.24, 1064.62, 2026.48, 1169.14, 2425.73, 2266.82, 893.285, 1299.6, 1615.69, 1955.45, 1084.31, 1546.11, 1529.82, 1816.24, 2148.28, 1410.36, 1552.85, 1781.22, 1780.3, 1697.19, 1190.53, 1069.78, 1108.17, 1851.27, 1342.98, 850.381, 1854.66, 1398.03, 1100.29, 2016.17, 1625.97, 1941.51, 701.989, 1930.6, 1708.51, 942.204, 1067.87, 709.937, 1600.57, 1412.42, 648.139, 1877.51, 885.259, 954.4, 997.229, 1723.12, 1855.66, 974.682, 1400.0, 753.804, 1554.74, 986.868, 1524.19, 1155.7]
  out "bin size":dbl=50.0
  in  "Min blockage (pA) 2":dbl format="%0.2f"
  in  "Max blockage (pA) 2":dbl=3000.0 format="%0.2f"
  in  "CUSUM levels histogram 2":bool=TRUE
  out "Scatter density":i32[][](graph)
  in  "Log t":bool=TRUE
  in  "Min I (pA)":dbl format="%_3g"
  in  "Max I (pA)":dbl=1.0 format="%_3g"
  in  "Current bins":i16=100
  in  "t Min (us)":dbl=1.0 format="%_3g"
  in  "t Max (us)":dbl=2000000.0 format="%_3g"
  in  "t Bins":i16=100
  out "Blockage vs Event time":cluster{"all rows":dbl[], "all rows":dbl[]}(graph)
  in  "Scatter plot":bool=TRUE
  in  "stop 2":bool
  in  "stop":bool
  in  "Dwell time min bin":dbl format="%0.2f"
  in  "Dwell time max bin":dbl=500.0 format="%0.2f"
  in  "Max block min (pA)":dbl format="%0.2f"
  in  "Max block max (pA)":dbl=1.0 format="%0.2f"
  in  "#bins (max block)":i32=50
  out "Max blockage (pA)":T1(graph)={"X Values"=[0.01, 0.03, 0.05, 0.07, 0.09, 0.11, 0.13, 0.15000000000000002, 0.16999999999999998, 0.19, 0.21000000000000002, 0.22999999999999998, 0.25, 0.27, 0.29000000000000004, 0.31, 0.33, 0.35, 0.37, 0.39, 0.41000000000000003, 0.43, 0.45, 0.47, 0.49, 0.51, 0.53, 0.55, 0.5700000000000001, 0.59, 0.61, 0.63, 0.65, 0.67, 0.6900000000000001, 0.71, 0.73, 0.75, 0.77, 0.79, 0.81, 0.8300000000000001, 0.85, 0.87, 0.89, 0.91, 0.93, 0.95, 0.97, 0.99], "Histogram: h(x)"=[0.0, 0.0, 0.0, 0.0, 0.0, 0.0, 0.0, 0.0024937655860349127, 0.0024937655860349127, 0.007481296758104738, 0.0024937655860349127, 0.02493765586034913, 0.03740648379052369, 0.032418952618453865, 0.04239401496259352, 0.032418952618453865, 0.03740648379052369, 0.032418952618453865, 0.022443890274314215, 0.057356608478802994, 0.02743142144638404, 0.0399002493765586, 0.022443890274314215, 0.029925187032418952, 0.04738154613466334, 0.03740648379052369, 0.032418952618453865, 0.02743142144638404, 0.032418952618453865, 0.014962593516209476, 0.029925187032418952, 0.032418952618453865, 0.03740648379052369, 0.08728179551122195, 0.05236907730673317, 0.02493765586034913, 0.007481296758104738, 0.02493765586034913, 0.012468827930174564, 0.007481296758104738, 0.012468827930174564, 0.0024937655860349127, 0.0024937655860349127, 0.017456359102244388, 0.0, 0.0, 0.0, 0.0, 0.0024937655860349127, 0.0]}
  out "Dwell time (us)":cluster{"Axis":dbl[], dbl[]}[](graph)=[{"Axis"=[5.0, 15.0, 25.0, 35.0, 45.0, 55.0, 65.0, 75.0, 85.0, 95.0, 105.0, 115.0, 125.0, 135.0, 145.0, 155.0, 165.0, 175.0, 185.0, 195.0, 205.0, 215.0, 225.0, 235.0, 245.0, 255.0, 265.0, 275.0, 285.0, 295.0, 305.0, 315.0, 325.0, 335.0, 345.0, 355.0, 365.0, 375.0, 385.0, 395.0, 405.0, 415.0, 425.0, 435.0, 445.0, 455.0, 465.0, 475.0, 485.0, 495.0], [47.0, 203.0, 25.0, 12.0, 11.0, 7.0, 6.0, 9.0, 7.0, 9.0, 2.0, 6.0, 5.0, 9.0, 0.0, 1.0, 4.0, 3.0, 3.0, 1.0, 0.0, 1.0, 0.0, 0.0, 1.0, 0.0, 0.0, 1.0, 1.0, 0.0, 0.0, 0.0, 0.0, 0.0, 1.0, 0.0, 0.0, 0.0, 0.0, 0.0, 0.0, 1.0, 0.0, 0.0, 0.0, 0.0, 1.0, 0.0, 1.0, 0.0]}, {"Axis"=[5.0, 15.0, 25.0, 35.0, 45.0, 55.0, 65.0, 75.0, 85.0, 95.0, 105.0, 115.0, 125.0, 135.0, 145.0, 155.0, 165.0, 175.0, 185.0, 195.0, 205.0, 215.0, 225.0, 235.0, 245.0, 255.0, 265.0, 275.0, 285.0, 295.0, 305.0, 315.0, 325.0, 335.0, 345.0, 355.0, 365.0, 375.0, 385.0, 395.0, 405.0, 415.0, 425.0, 435.0, 445.0, 455.0, 465.0, 475.0, 485.0, 495.0], [0.12433862433862433, 0.5370370370370371, 0.06613756613756613, 0.031746031746031744, 0.0291005291005291, 0.018518518518518517, 0.015873015873015872, 0.023809523809523808, 0.018518518518518517, 0.023809523809523808, 0.005291005291005291, 0.015873015873015872, 0.013227513227513227, 0.023809523809523808, 0.0, 0.0026455026455026454, 0.010582010582010581, 0.007936507936507936, 0.007936507936507936, 0.0026455026455026454, 0.0, 0.0026455026455026454, 0.0, 0.0, 0.0026455026455026454, 0.0, 0.0, 0.0026455026455026454, 0.0026455026455026454, 0.0, 0.0, 0.0, 0.0, 0.0, 0.0026455026455026454, 0.0, 0.0, 0.0, 0.0, 0.0, 0.0, 0.0026455026455026454, 0.0, 0.0, 0.0, 0.0, 0.0026455026455026454, 0.0, 0.0026455026455026454, 0.0]}]
  out "min dwell time":dbl=4.0
  out "max dwell time":dbl=1180000.0
  in  "#bins (dwell)":i32=50
  in  "Max blockage histogram":bool=TRUE
  in  "Dwell time histogram":bool=TRUE
  out "Events analysed":i32
  out "sum (dummy check)":dbl=0.9963822472223787
  out "event length":i32=216
  out "Histogram":i32[](array[numeric])=[0, 0, 0, 0, 0, 0, 0, 0, 0, 0, 0, 1, 0, 0, 0, 0, 0, 0, 0, 0, 0, 0, 0, 0, 0, 0, 0, 0, 0, 0, 0, 0, 0, 0, 0, 0, 0, 0, 0, 0, 0, 0, 0, 0, 0, 0, 0, 0, 0, 0]
  out "Levels histogram":cluster{"Axis":dbl[], dbl[]}(graph)={"Axis"=[-3465.0, -3395.0, -3325.0, -3255.0, -3185.0, -3115.0, -3045.0, -2975.0, -2905.0, -2835.0, -2765.0, -2695.0, -2625.0, -2555.0, -2485.0, -2415.0, -2345.0, -2275.0, -2205.0, -2135.0, -2065.0, -1995.0, -1925.0, -1855.0, -1785.0, -1715.0, -1645.0, -1575.0, -1505.0, -1435.0, -1365.0, -1295.0, -1225.0, -1155.0, -1085.0, -1015.0, -945.0, -875.0, -805.0, -735.0, -665.0, -595.0, -525.0, -455.0, -385.0, -315.0, -245.0, -175.0, -105.0, -35.0], [0.0004949710534058188, 0.0005575107571682827, 0.0001833475976425106, 0.00031649062619960714, 0.0009038635940800331, 0.0009151745206729308, 0.0008976400417446829, 0.0016365757773167046, 0.0033132967394204757, 0.005761032897407708, 0.025661984455272346, 0.3536324808135091, 0.4010886480266952, 0.04444740968906965, 0.00610171878792866, 0.001842720890428927, 0.0011289414947405505, 0.0008389566023915335, 0.0011172240577151799, 0.0005197184732067511, 0.0006034201729588347, 0.0004933665394832644, 0.00032185808538917843, 0.0006615560073560593, 0.0005686703564385492, 0.0009888549020411514, 0.0007824467779992721, 0.0016983786202295686, 0.0020475788830917017, 0.0015802329978052941, 0.005471286054086217, 0.006872608057804315, 0.0025711244937169754, 0.006312800625638749, 0.00696186076810715, 0.006686656172749102, 0.011719105900513196, 0.03457162380260294, 0.025076556913255776, 0.005739451255138987, 0.006988723622568358, 0.0054167527145173285, 0.003024455202881837, 0.004714153538480746, 0.0017621018281088823, 0.001344500548197642, 1.1613322803920659e-05, 0.0, 1.1446624390467251e-05, 1.935553800653443e-05]}
  out "Cumulative histogram":i32[](array[numeric])
  in  "# bins":i32=60
  in  "Min current (pA)":dbl=-3500.0 format="%0.2f"
  in  "Max current (pA)":dbl format="%0.2f"
  in  "CUSUM levels histogram":bool
  out "Event details":dbl[](array[numeric])=[5.231562, 144932.0, 2413.94, 26.0] caption="Time (s)\n      Length (us)\nMax block (pA)   \n           # levels"
  out "CUSUM event":path=path "D:/DATA/2015/Sep2015/sep22/1705_10111_36MLiClpH8_3uLlane1dsDNA_150mV/events/event_00000.csv"
  out "CUSUM event":cluster{"Y":dbl[], "Y":dbl[]}[](graph)
  in  "Event Index":i32
  out "All Files in Dir":path[](array[path])=[path "D:/DATA/2015/Sep2015/sep22/1705_10111_36MLiClpH8_3uLlane1dsDNA_150mV/events/event_00000.csv", path "D:/DATA/2015/Sep2015/sep22/1705_10111_36MLiClpH8_3uLlane1dsDNA_150mV/events/event_00002.csv", path "D:/DATA/2015/Sep2015/sep22/1705_10111_36MLiClpH8_3uLlane1dsDNA_150mV/events/event_00003.csv", path "D:/DATA/2015/Sep2015/sep22/1705_10111_36MLiClpH8_3uLlane1dsDNA_150mV/events/event_00004.csv", path "D:/DATA/2015/Sep2015/sep22/1705_10111_36MLiClpH8_3uLlane1dsDNA_150mV/events/event_00005.csv", path "D:/DATA/2015/Sep2015/sep22/1705_10111_36MLiClpH8_3uLlane1dsDNA_150mV/events/event_00006.csv", path "D:/DATA/2015/Sep2015/sep22/1705_10111_36MLiClpH8_3uLlane1dsDNA_150mV/events/event_00009.csv", path "D:/DATA/2015/Sep2015/sep22/1705_10111_36MLiClpH8_3uLlane1dsDNA_150mV/events/event_00010.csv", path "D:/DATA/2015/Sep2015/sep22/1705_10111_36MLiClpH8_3uLlane1dsDNA_150mV/events/event_00011.csv", path "D:/DATA/2015/Sep2015/sep22/1705_10111_36MLiClpH8_3uLlane1dsDNA_150mV/events/event_00013.csv", path "D:/DATA/2015/Sep2015/sep22/1705_10111_36MLiClpH8_3uLlane1dsDNA_150mV/events/event_00015.csv", path "D:/DATA/2015/Sep2015/sep22/1705_10111_36MLiClpH8_3uLlane1dsDNA_150mV/events/event_00016.csv", path "D:/DATA/2015/Sep2015/sep22/1705_10111_36MLiClpH8_3uLlane1dsDNA_150mV/events/event_00017.csv", path "D:/DATA/2015/Sep2015/sep22/1705_10111_36MLiClpH8_3uLlane1dsDNA_150mV/events/event_00018.csv", path "D:/DATA/2015/Sep2015/sep22/1705_10111_36MLiClpH8_3uLlane1dsDNA_150mV/events/event_00020.csv", path "D:/DATA/2015/Sep2015/sep22/1705_10111_36MLiClpH8_3uLlane1dsDNA_150mV/events/event_00025.csv", path "D:/DATA/2015/Sep2015/sep22/1705_10111_36MLiClpH8_3uLlane1dsDNA_150mV/events/event_00026.csv", path "D:/DATA/2015/Sep2015/sep22/1705_10111_36MLiClpH8_3uLlane1dsDNA_150mV/events/event_00027.csv", path "D:/DATA/2015/Sep2015/sep22/1705_10111_36MLiClpH8_3uLlane1dsDNA_150mV/events/event_00028.csv", path "D:/DATA/2015/Sep2015/sep22/1705_10111_36MLiClpH8_3uLlane1dsDNA_150mV/events/event_00029.csv", path "D:/DATA/2015/Sep2015/sep22/1705_10111_36MLiClpH8_3uLlane1dsDNA_150mV/events/event_00031.csv", path "D:/DATA/2015/Sep2015/sep22/1705_10111_36MLiClpH8_3uLlane1dsDNA_150mV/events/event_00032.csv", path "D:/DATA/2015/Sep2015/sep22/1705_10111_36MLiClpH8_3uLlane1dsDNA_150mV/events/event_00033.csv", path "D:/DATA/2015/Sep2015/sep22/1705_10111_36MLiClpH8_3uLlane1dsDNA_150mV/events/event_00036.csv", path "D:/DATA/2015/Sep2015/sep22/1705_10111_36MLiClpH8_3uLlane1dsDNA_150mV/events/event_00038.csv", path "D:/DATA/2015/Sep2015/sep22/1705_10111_36MLiClpH8_3uLlane1dsDNA_150mV/events/event_00040.csv", path "D:/DATA/2015/Sep2015/sep22/1705_10111_36MLiClpH8_3uLlane1dsDNA_150mV/events/event_00041.csv", path "D:/DATA/2015/Sep2015/sep22/1705_10111_36MLiClpH8_3uLlane1dsDNA_150mV/events/event_00043.csv", path "D:/DATA/2015/Sep2015/sep22/1705_10111_36MLiClpH8_3uLlane1dsDNA_150mV/events/event_00044.csv", path "D:/DATA/2015/Sep2015/sep22/1705_10111_36MLiClpH8_3uLlane1dsDNA_150mV/events/event_00045.csv", path "D:/DATA/2015/Sep2015/sep22/1705_10111_36MLiClpH8_3uLlane1dsDNA_150mV/events/event_00056.csv", path "D:/DATA/2015/Sep2015/sep22/1705_10111_36MLiClpH8_3uLlane1dsDNA_150mV/events/event_00057.csv", path "D:/DATA/2015/Sep2015/sep22/1705_10111_36MLiClpH8_3uLlane1dsDNA_150mV/events/event_00058.csv", path "D:/DATA/2015/Sep2015/sep22/1705_10111_36MLiClpH8_3uLlane1dsDNA_150mV/events/event_00060.csv", path "D:/DATA/2015/Sep2015/sep22/1705_10111_36MLiClpH8_3uLlane1dsDNA_150mV/events/event_00062.csv", path "D:/DATA/2015/Sep2015/sep22/1705_10111_36MLiClpH8_3uLlane1dsDNA_150mV/events/event_00065.csv", path "D:/DATA/2015/Sep2015/sep22/1705_10111_36MLiClpH8_3uLlane1dsDNA_150mV/events/event_00066.csv", path "D:/DATA/2015/Sep2015/sep22/1705_10111_36MLiClpH8_3uLlane1dsDNA_150mV/events/event_00067.csv", path "D:/DATA/2015/Sep2015/sep22/1705_10111_36MLiClpH8_3uLlane1dsDNA_150mV/events/event_00068.csv", path "D:/DATA/2015/Sep2015/sep22/1705_10111_36MLiClpH8_3uLlane1dsDNA_150mV/events/event_00069.csv", path "D:/DATA/2015/Sep2015/sep22/1705_10111_36MLiClpH8_3uLlane1dsDNA_150mV/events/event_00070.csv", path "D:/DATA/2015/Sep2015/sep22/1705_10111_36MLiClpH8_3uLlane1dsDNA_150mV/events/event_00071.csv", path "D:/DATA/2015/Sep2015/sep22/1705_10111_36MLiClpH8_3uLlane1dsDNA_150mV/events/event_00072.csv", path "D:/DATA/2015/Sep2015/sep22/1705_10111_36MLiClpH8_3uLlane1dsDNA_150mV/events/event_00073.csv", path "D:/DATA/2015/Sep2015/sep22/1705_10111_36MLiClpH8_3uLlane1dsDNA_150mV/events/event_00074.csv", path "D:/DATA/2015/Sep2015/sep22/1705_10111_36MLiClpH8_3uLlane1dsDNA_150mV/events/event_00075.csv", path "D:/DATA/2015/Sep2015/sep22/1705_10111_36MLiClpH8_3uLlane1dsDNA_150mV/events/event_00076.csv", path "D:/DATA/2015/Sep2015/sep22/1705_10111_36MLiClpH8_3uLlane1dsDNA_150mV/events/event_00077.csv", path "D:/DATA/2015/Sep2015/sep22/1705_10111_36MLiClpH8_3uLlane1dsDNA_150mV/events/event_00078.csv", path "D:/DATA/2015/Sep2015/sep22/1705_10111_36MLiClpH8_3uLlane1dsDNA_150mV/events/event_00079.csv", path "D:/DATA/2015/Sep2015/sep22/1705_10111_36MLiClpH8_3uLlane1dsDNA_150mV/events/event_00081.csv", path "D:/DATA/2015/Sep2015/sep22/1705_10111_36MLiClpH8_3uLlane1dsDNA_150mV/events/event_00082.csv", path "D:/DATA/2015/Sep2015/sep22/1705_10111_36MLiClpH8_3uLlane1dsDNA_150mV/events/event_00085.csv", path "D:/DATA/2015/Sep2015/sep22/1705_10111_36MLiClpH8_3uLlane1dsDNA_150mV/events/event_00086.csv", path "D:/DATA/2015/Sep2015/sep22/1705_10111_36MLiClpH8_3uLlane1dsDNA_150mV/events/event_00087.csv", path "D:/DATA/2015/Sep2015/sep22/1705_10111_36MLiClpH8_3uLlane1dsDNA_150mV/events/event_00088.csv", path "D:/DATA/2015/Sep2015/sep22/1705_10111_36MLiClpH8_3uLlane1dsDNA_150mV/events/event_00089.csv", path "D:/DATA/2015/Sep2015/sep22/1705_10111_36MLiClpH8_3uLlane1dsDNA_150mV/events/event_00091.csv", path "D:/DATA/2015/Sep2015/sep22/1705_10111_36MLiClpH8_3uLlane1dsDNA_150mV/events/event_00092.csv", path "D:/DATA/2015/Sep2015/sep22/1705_10111_36MLiClpH8_3uLlane1dsDNA_150mV/events/event_00094.csv", path "D:/DATA/2015/Sep2015/sep22/1705_10111_36MLiClpH8_3uLlane1dsDNA_150mV/events/event_00095.csv", path "D:/DATA/2015/Sep2015/sep22/1705_10111_36MLiClpH8_3uLlane1dsDNA_150mV/events/event_00096.csv", path "D:/DATA/2015/Sep2015/sep22/1705_10111_36MLiClpH8_3uLlane1dsDNA_150mV/events/event_00098.csv", path "D:/DATA/2015/Sep2015/sep22/1705_10111_36MLiClpH8_3uLlane1dsDNA_150mV/events/event_00099.csv", path "D:/DATA/2015/Sep2015/sep22/1705_10111_36MLiClpH8_3uLlane1dsDNA_150mV/events/event_00100.csv", path "D:/DATA/2015/Sep2015/sep22/1705_10111_36MLiClpH8_3uLlane1dsDNA_150mV/events/event_00101.csv", path "D:/DATA/2015/Sep2015/sep22/1705_10111_36MLiClpH8_3uLlane1dsDNA_150mV/events/event_00102.csv", path "D:/DATA/2015/Sep2015/sep22/1705_10111_36MLiClpH8_3uLlane1dsDNA_150mV/events/event_00103.csv", path "D:/DATA/2015/Sep2015/sep22/1705_10111_36MLiClpH8_3uLlane1dsDNA_150mV/events/event_00104.csv", path "D:/DATA/2015/Sep2015/sep22/1705_10111_36MLiClpH8_3uLlane1dsDNA_150mV/events/event_00106.csv", path "D:/DATA/2015/Sep2015/sep22/1705_10111_36MLiClpH8_3uLlane1dsDNA_150mV/events/event_00107.csv", path "D:/DATA/2015/Sep2015/sep22/1705_10111_36MLiClpH8_3uLlane1dsDNA_150mV/events/event_00109.csv", path "D:/DATA/2015/Sep2015/sep22/1705_10111_36MLiClpH8_3uLlane1dsDNA_150mV/events/event_00110.csv", path "D:/DATA/2015/Sep2015/sep22/1705_10111_36MLiClpH8_3uLlane1dsDNA_150mV/events/event_00112.csv", path "D:/DATA/2015/Sep2015/sep22/1705_10111_36MLiClpH8_3uLlane1dsDNA_150mV/events/event_00113.csv", path "D:/DATA/2015/Sep2015/sep22/1705_10111_36MLiClpH8_3uLlane1dsDNA_150mV/events/event_00114.csv", path "D:/DATA/2015/Sep2015/sep22/1705_10111_36MLiClpH8_3uLlane1dsDNA_150mV/events/event_00116.csv", path "D:/DATA/2015/Sep2015/sep22/1705_10111_36MLiClpH8_3uLlane1dsDNA_150mV/events/event_00117.csv", path "D:/DATA/2015/Sep2015/sep22/1705_10111_36MLiClpH8_3uLlane1dsDNA_150mV/events/event_00118.csv", path "D:/DATA/2015/Sep2015/sep22/1705_10111_36MLiClpH8_3uLlane1dsDNA_150mV/events/event_00119.csv", path "D:/DATA/2015/Sep2015/sep22/1705_10111_36MLiClpH8_3uLlane1dsDNA_150mV/events/event_00120.csv", path "D:/DATA/2015/Sep2015/sep22/1705_10111_36MLiClpH8_3uLlane1dsDNA_150mV/events/event_00121.csv", path "D:/DATA/2015/Sep2015/sep22/1705_10111_36MLiClpH8_3uLlane1dsDNA_150mV/events/event_00122.csv", path "D:/DATA/2015/Sep2015/sep22/1705_10111_36MLiClpH8_3uLlane1dsDNA_150mV/events/event_00123.csv", path "D:/DATA/2015/Sep2015/sep22/1705_10111_36MLiClpH8_3uLlane1dsDNA_150mV/events/event_00125.csv", path "D:/DATA/2015/Sep2015/sep22/1705_10111_36MLiClpH8_3uLlane1dsDNA_150mV/events/event_00126.csv", path "D:/DATA/2015/Sep2015/sep22/1705_10111_36MLiClpH8_3uLlane1dsDNA_150mV/events/event_00127.csv", path "D:/DATA/2015/Sep2015/sep22/1705_10111_36MLiClpH8_3uLlane1dsDNA_150mV/events/event_00128.csv", path "D:/DATA/2015/Sep2015/sep22/1705_10111_36MLiClpH8_3uLlane1dsDNA_150mV/events/event_00129.csv", path "D:/DATA/2015/Sep2015/sep22/1705_10111_36MLiClpH8_3uLlane1dsDNA_150mV/events/event_00131.csv", path "D:/DATA/2015/Sep2015/sep22/1705_10111_36MLiClpH8_3uLlane1dsDNA_150mV/events/event_00132.csv", path "D:/DATA/2015/Sep2015/sep22/1705_10111_36MLiClpH8_3uLlane1dsDNA_150mV/events/event_00133.csv", path "D:/DATA/2015/Sep2015/sep22/1705_10111_36MLiClpH8_3uLlane1dsDNA_150mV/events/event_00134.csv", path "D:/DATA/2015/Sep2015/sep22/1705_10111_36MLiClpH8_3uLlane1dsDNA_150mV/events/event_00135.csv", path "D:/DATA/2015/Sep2015/sep22/1705_10111_36MLiClpH8_3uLlane1dsDNA_150mV/events/event_00136.csv", path "D:/DATA/2015/Sep2015/sep22/1705_10111_36MLiClpH8_3uLlane1dsDNA_150mV/events/event_00138.csv", path "D:/DATA/2015/Sep2015/sep22/1705_10111_36MLiClpH8_3uLlane1dsDNA_150mV/events/event_00139.csv", path "D:/DATA/2015/Sep2015/sep22/1705_10111_36MLiClpH8_3uLlane1dsDNA_150mV/events/event_00140.csv", path "D:/DATA/2015/Sep2015/sep22/1705_10111_36MLiClpH8_3uLlane1dsDNA_150mV/events/event_00141.csv", path "D:/DATA/2015/Sep2015/sep22/1705_10111_36MLiClpH8_3uLlane1dsDNA_150mV/events/event_00142.csv", path "D:/DATA/2015/Sep2015/sep22/1705_10111_36MLiClpH8_3uLlane1dsDNA_150mV/events/event_00143.csv", path "D:/DATA/2015/Sep2015/sep22/1705_10111_36MLiClpH8_3uLlane1dsDNA_150mV/events/event_00144.csv", path "D:/DATA/2015/Sep2015/sep22/1705_10111_36MLiClpH8_3uLlane1dsDNA_150mV/events/event_00145.csv", path "D:/DATA/2015/Sep2015/sep22/1705_10111_36MLiClpH8_3uLlane1dsDNA_150mV/events/event_00147.csv", path "D:/DATA/2015/Sep2015/sep22/1705_10111_36MLiClpH8_3uLlane1dsDNA_150mV/events/event_00149.csv", path "D:/DATA/2015/Sep2015/sep22/1705_10111_36MLiClpH8_3uLlane1dsDNA_150mV/events/event_00150.csv", path "D:/DATA/2015/Sep2015/sep22/1705_10111_36MLiClpH8_3uLlane1dsDNA_150mV/events/event_00151.csv", path "D:/DATA/2015/Sep2015/sep22/1705_10111_36MLiClpH8_3uLlane1dsDNA_150mV/events/event_00152.csv", path "D:/DATA/2015/Sep2015/sep22/1705_10111_36MLiClpH8_3uLlane1dsDNA_150mV/events/event_00153.csv", path "D:/DATA/2015/Sep2015/sep22/1705_10111_36MLiClpH8_3uLlane1dsDNA_150mV/events/event_00155.csv", path "D:/DATA/2015/Sep2015/sep22/1705_10111_36MLiClpH8_3uLlane1dsDNA_150mV/events/event_00157.csv", path "D:/DATA/2015/Sep2015/sep22/1705_10111_36MLiClpH8_3uLlane1dsDNA_150mV/events/event_00159.csv", path "D:/DATA/2015/Sep2015/sep22/1705_10111_36MLiClpH8_3uLlane1dsDNA_150mV/events/event_00160.csv", path "D:/DATA/2015/Sep2015/sep22/1705_10111_36MLiClpH8_3uLlane1dsDNA_150mV/events/event_00161.csv", path "D:/DATA/2015/Sep2015/sep22/1705_10111_36MLiClpH8_3uLlane1dsDNA_150mV/events/event_00162.csv", path "D:/DATA/2015/Sep2015/sep22/1705_10111_36MLiClpH8_3uLlane1dsDNA_150mV/events/event_00163.csv", path "D:/DATA/2015/Sep2015/sep22/1705_10111_36MLiClpH8_3uLlane1dsDNA_150mV/events/event_00164.csv", path "D:/DATA/2015/Sep2015/sep22/1705_10111_36MLiClpH8_3uLlane1dsDNA_150mV/events/event_00165.csv", path "D:/DATA/2015/Sep2015/sep22/1705_10111_36MLiClpH8_3uLlane1dsDNA_150mV/events/event_00166.csv", path "D:/DATA/2015/Sep2015/sep22/1705_10111_36MLiClpH8_3uLlane1dsDNA_150mV/events/event_00167.csv", path "D:/DATA/2015/Sep2015/sep22/1705_10111_36MLiClpH8_3uLlane1dsDNA_150mV/events/event_00168.csv", path "D:/DATA/2015/Sep2015/sep22/1705_10111_36MLiClpH8_3uLlane1dsDNA_150mV/events/event_00169.csv", path "D:/DATA/2015/Sep2015/sep22/1705_10111_36MLiClpH8_3uLlane1dsDNA_150mV/events/event_00170.csv", path "D:/DATA/2015/Sep2015/sep22/1705_10111_36MLiClpH8_3uLlane1dsDNA_150mV/events/event_00171.csv", path "D:/DATA/2015/Sep2015/sep22/1705_10111_36MLiClpH8_3uLlane1dsDNA_150mV/events/event_00172.csv", path "D:/DATA/2015/Sep2015/sep22/1705_10111_36MLiClpH8_3uLlane1dsDNA_150mV/events/event_00174.csv", path "D:/DATA/2015/Sep2015/sep22/1705_10111_36MLiClpH8_3uLlane1dsDNA_150mV/events/event_00177.csv", path "D:/DATA/2015/Sep2015/sep22/1705_10111_36MLiClpH8_3uLlane1dsDNA_150mV/events/event_00179.csv", path "D:/DATA/2015/Sep2015/sep22/1705_10111_36MLiClpH8_3uLlane1dsDNA_150mV/events/event_00180.csv", path "D:/DATA/2015/Sep2015/sep22/1705_10111_36MLiClpH8_3uLlane1dsDNA_150mV/events/event_00183.csv", path "D:/DATA/2015/Sep2015/sep22/1705_10111_36MLiClpH8_3uLlane1dsDNA_150mV/events/event_00184.csv", path "D:/DATA/2015/Sep2015/sep22/1705_10111_36MLiClpH8_3uLlane1dsDNA_150mV/events/event_00185.csv", path "D:/DATA/2015/Sep2015/sep22/1705_10111_36MLiClpH8_3uLlane1dsDNA_150mV/events/event_00186.csv", path "D:/DATA/2015/Sep2015/sep22/1705_10111_36MLiClpH8_3uLlane1dsDNA_150mV/events/event_00187.csv", path "D:/DATA/2015/Sep2015/sep22/1705_10111_36MLiClpH8_3uLlane1dsDNA_150mV/events/event_00189.csv", path "D:/DATA/2015/Sep2015/sep22/1705_10111_36MLiClpH8_3uLlane1dsDNA_150mV/events/event_00190.csv", path "D:/DATA/2015/Sep2015/sep22/1705_10111_36MLiClpH8_3uLlane1dsDNA_150mV/events/event_00194.csv", path "D:/DATA/2015/Sep2015/sep22/1705_10111_36MLiClpH8_3uLlane1dsDNA_150mV/events/event_00196.csv", path "D:/DATA/2015/Sep2015/sep22/1705_10111_36MLiClpH8_3uLlane1dsDNA_150mV/events/event_00197.csv", path "D:/DATA/2015/Sep2015/sep22/1705_10111_36MLiClpH8_3uLlane1dsDNA_150mV/events/event_00198.csv", path "D:/DATA/2015/Sep2015/sep22/1705_10111_36MLiClpH8_3uLlane1dsDNA_150mV/events/event_00199.csv", path "D:/DATA/2015/Sep2015/sep22/1705_10111_36MLiClpH8_3uLlane1dsDNA_150mV/events/event_00200.csv", path "D:/DATA/2015/Sep2015/sep22/1705_10111_36MLiClpH8_3uLlane1dsDNA_150mV/events/event_00201.csv", path "D:/DATA/2015/Sep2015/sep22/1705_10111_36MLiClpH8_3uLlane1dsDNA_150mV/events/event_00202.csv", path "D:/DATA/2015/Sep2015/sep22/1705_10111_36MLiClpH8_3uLlane1dsDNA_150mV/events/event_00205.csv", path "D:/DATA/2015/Sep2015/sep22/1705_10111_36MLiClpH8_3uLlane1dsDNA_150mV/events/event_00206.csv", path "D:/DATA/2015/Sep2015/sep22/1705_10111_36MLiClpH8_3uLlane1dsDNA_150mV/events/event_00207.csv", path "D:/DATA/2015/Sep2015/sep22/1705_10111_36MLiClpH8_3uLlane1dsDNA_150mV/events/event_00208.csv", path "D:/DATA/2015/Sep2015/sep22/1705_10111_36MLiClpH8_3uLlane1dsDNA_150mV/events/event_00209.csv", path "D:/DATA/2015/Sep2015/sep22/1705_10111_36MLiClpH8_3uLlane1dsDNA_150mV/events/event_00210.csv", path "D:/DATA/2015/Sep2015/sep22/1705_10111_36MLiClpH8_3uLlane1dsDNA_150mV/events/event_00211.csv", path "D:/DATA/2015/Sep2015/sep22/1705_10111_36MLiClpH8_3uLlane1dsDNA_150mV/events/event_00212.csv", path "D:/DATA/2015/Sep2015/sep22/1705_10111_36MLiClpH8_3uLlane1dsDNA_150mV/events/event_00213.csv", path "D:/DATA/2015/Sep2015/sep22/1705_10111_36MLiClpH8_3uLlane1dsDNA_150mV/events/event_00214.csv", path "D:/DATA/2015/Sep2015/sep22/1705_10111_36MLiClpH8_3uLlane1dsDNA_150mV/events/event_00215.csv", path "D:/DATA/2015/Sep2015/sep22/1705_10111_36MLiClpH8_3uLlane1dsDNA_150mV/events/event_00216.csv", path "D:/DATA/2015/Sep2015/sep22/1705_10111_36MLiClpH8_3uLlane1dsDNA_150mV/events/event_00217.csv", path "D:/DATA/2015/Sep2015/sep22/1705_10111_36MLiClpH8_3uLlane1dsDNA_150mV/events/event_00218.csv", path "D:/DATA/2015/Sep2015/sep22/1705_10111_36MLiClpH8_3uLlane1dsDNA_150mV/events/event_00219.csv", path "D:/DATA/2015/Sep2015/sep22/1705_10111_36MLiClpH8_3uLlane1dsDNA_150mV/events/event_00221.csv", path "D:/DATA/2015/Sep2015/sep22/1705_10111_36MLiClpH8_3uLlane1dsDNA_150mV/events/event_00223.csv", path "D:/DATA/2015/Sep2015/sep22/1705_10111_36MLiClpH8_3uLlane1dsDNA_150mV/events/event_00224.csv", path "D:/DATA/2015/Sep2015/sep22/1705_10111_36MLiClpH8_3uLlane1dsDNA_150mV/events/event_00225.csv", path "D:/DATA/2015/Sep2015/sep22/1705_10111_36MLiClpH8_3uLlane1dsDNA_150mV/events/event_00226.csv", path "D:/DATA/2015/Sep2015/sep22/1705_10111_36MLiClpH8_3uLlane1dsDNA_150mV/events/event_00227.csv", path "D:/DATA/2015/Sep2015/sep22/1705_10111_36MLiClpH8_3uLlane1dsDNA_150mV/events/event_00228.csv", path "D:/DATA/2015/Sep2015/sep22/1705_10111_36MLiClpH8_3uLlane1dsDNA_150mV/events/event_00229.csv", path "D:/DATA/2015/Sep2015/sep22/1705_10111_36MLiClpH8_3uLlane1dsDNA_150mV/events/event_00230.csv", path "D:/DATA/2015/Sep2015/sep22/1705_10111_36MLiClpH8_3uLlane1dsDNA_150mV/events/event_00231.csv", path "D:/DATA/2015/Sep2015/sep22/1705_10111_36MLiClpH8_3uLlane1dsDNA_150mV/events/event_00232.csv", path "D:/DATA/2015/Sep2015/sep22/1705_10111_36MLiClpH8_3uLlane1dsDNA_150mV/events/event_00233.csv", path "D:/DATA/2015/Sep2015/sep22/1705_10111_36MLiClpH8_3uLlane1dsDNA_150mV/events/event_00234.csv", path "D:/DATA/2015/Sep2015/sep22/1705_10111_36MLiClpH8_3uLlane1dsDNA_150mV/events/event_00235.csv", path "D:/DATA/2015/Sep2015/sep22/1705_10111_36MLiClpH8_3uLlane1dsDNA_150mV/events/event_00236.csv", path "D:/DATA/2015/Sep2015/sep22/1705_10111_36MLiClpH8_3uLlane1dsDNA_150mV/events/event_00237.csv", path "D:/DATA/2015/Sep2015/sep22/1705_10111_36MLiClpH8_3uLlane1dsDNA_150mV/events/event_00238.csv", path "D:/DATA/2015/Sep2015/sep22/1705_10111_36MLiClpH8_3uLlane1dsDNA_150mV/events/event_00239.csv", path "D:/DATA/2015/Sep2015/sep22/1705_10111_36MLiClpH8_3uLlane1dsDNA_150mV/events/event_00241.csv", path "D:/DATA/2015/Sep2015/sep22/1705_10111_36MLiClpH8_3uLlane1dsDNA_150mV/events/event_00243.csv", path "D:/DATA/2015/Sep2015/sep22/1705_10111_36MLiClpH8_3uLlane1dsDNA_150mV/events/event_00244.csv", path "D:/DATA/2015/Sep2015/sep22/1705_10111_36MLiClpH8_3uLlane1dsDNA_150mV/events/event_00245.csv", path "D:/DATA/2015/Sep2015/sep22/1705_10111_36MLiClpH8_3uLlane1dsDNA_150mV/events/event_00246.csv", path "D:/DATA/2015/Sep2015/sep22/1705_10111_36MLiClpH8_3uLlane1dsDNA_150mV/events/event_00247.csv", path "D:/DATA/2015/Sep2015/sep22/1705_10111_36MLiClpH8_3uLlane1dsDNA_150mV/events/event_00248.csv", path "D:/DATA/2015/Sep2015/sep22/1705_10111_36MLiClpH8_3uLlane1dsDNA_150mV/events/event_00249.csv", path "D:/DATA/2015/Sep2015/sep22/1705_10111_36MLiClpH8_3uLlane1dsDNA_150mV/events/event_00250.csv", path "D:/DATA/2015/Sep2015/sep22/1705_10111_36MLiClpH8_3uLlane1dsDNA_150mV/events/event_00251.csv", path "D:/DATA/2015/Sep2015/sep22/1705_10111_36MLiClpH8_3uLlane1dsDNA_150mV/events/event_00253.csv", path "D:/DATA/2015/Sep2015/sep22/1705_10111_36MLiClpH8_3uLlane1dsDNA_150mV/events/event_00254.csv", path "D:/DATA/2015/Sep2015/sep22/1705_10111_36MLiClpH8_3uLlane1dsDNA_150mV/events/event_00255.csv", path "D:/DATA/2015/Sep2015/sep22/1705_10111_36MLiClpH8_3uLlane1dsDNA_150mV/events/event_00256.csv", path "D:/DATA/2015/Sep2015/sep22/1705_10111_36MLiClpH8_3uLlane1dsDNA_150mV/events/event_00257.csv", path "D:/DATA/2015/Sep2015/sep22/1705_10111_36MLiClpH8_3uLlane1dsDNA_150mV/events/event_00258.csv", path "D:/DATA/2015/Sep2015/sep22/1705_10111_36MLiClpH8_3uLlane1dsDNA_150mV/events/event_00261.csv", path "D:/DATA/2015/Sep2015/sep22/1705_10111_36MLiClpH8_3uLlane1dsDNA_150mV/events/event_00262.csv", path "D:/DATA/2015/Sep2015/sep22/1705_10111_36MLiClpH8_3uLlane1dsDNA_150mV/events/event_00264.csv", path "D:/DATA/2015/Sep2015/sep22/1705_10111_36MLiClpH8_3uLlane1dsDNA_150mV/events/event_00265.csv", path "D:/DATA/2015/Sep2015/sep22/1705_10111_36MLiClpH8_3uLlane1dsDNA_150mV/events/event_00266.csv", path "D:/DATA/2015/Sep2015/sep22/1705_10111_36MLiClpH8_3uLlane1dsDNA_150mV/events/event_00267.csv", path "D:/DATA/2015/Sep2015/sep22/1705_10111_36MLiClpH8_3uLlane1dsDNA_150mV/events/event_00269.csv", path "D:/DATA/2015/Sep2015/sep22/1705_10111_36MLiClpH8_3uLlane1dsDNA_150mV/events/event_00270.csv", path "D:/DATA/2015/Sep2015/sep22/1705_10111_36MLiClpH8_3uLlane1dsDNA_150mV/events/event_00271.csv", path "D:/DATA/2015/Sep2015/sep22/1705_10111_36MLiClpH8_3uLlane1dsDNA_150mV/events/event_00272.csv", path "D:/DATA/2015/Sep2015/sep22/1705_10111_36MLiClpH8_3uLlane1dsDNA_150mV/events/event_00273.csv", path "D:/DATA/2015/Sep2015/sep22/1705_10111_36MLiClpH8_3uLlane1dsDNA_150mV/events/event_00275.csv", path "D:/DATA/2015/Sep2015/sep22/1705_10111_36MLiClpH8_3uLlane1dsDNA_150mV/events/event_00276.csv", path "D:/DATA/2015/Sep2015/sep22/1705_10111_36MLiClpH8_3uLlane1dsDNA_150mV/events/event_00277.csv", path "D:/DATA/2015/Sep2015/sep22/1705_10111_36MLiClpH8_3uLlane1dsDNA_150mV/events/event_00278.csv", path "D:/DATA/2015/Sep2015/sep22/1705_10111_36MLiClpH8_3uLlane1dsDNA_150mV/events/event_00280.csv", path "D:/DATA/2015/Sep2015/sep22/1705_10111_36MLiClpH8_3uLlane1dsDNA_150mV/events/event_00283.csv", path "D:/DATA/2015/Sep2015/sep22/1705_10111_36MLiClpH8_3uLlane1dsDNA_150mV/events/event_00285.csv", path "D:/DATA/2015/Sep2015/sep22/1705_10111_36MLiClpH8_3uLlane1dsDNA_150mV/events/event_00289.csv", path "D:/DATA/2015/Sep2015/sep22/1705_10111_36MLiClpH8_3uLlane1dsDNA_150mV/events/event_00290.csv", path "D:/DATA/2015/Sep2015/sep22/1705_10111_36MLiClpH8_3uLlane1dsDNA_150mV/events/event_00292.csv", path "D:/DATA/2015/Sep2015/sep22/1705_10111_36MLiClpH8_3uLlane1dsDNA_150mV/events/event_00293.csv", path "D:/DATA/2015/Sep2015/sep22/1705_10111_36MLiClpH8_3uLlane1dsDNA_150mV/events/event_00295.csv", path "D:/DATA/2015/Sep2015/sep22/1705_10111_36MLiClpH8_3uLlane1dsDNA_150mV/events/event_00296.csv", path "D:/DATA/2015/Sep2015/sep22/1705_10111_36MLiClpH8_3uLlane1dsDNA_150mV/events/event_00297.csv", path "D:/DATA/2015/Sep2015/sep22/1705_10111_36MLiClpH8_3uLlane1dsDNA_150mV/events/event_00298.csv", path "D:/DATA/2015/Sep2015/sep22/1705_10111_36MLiClpH8_3uLlane1dsDNA_150mV/events/event_00299.csv", path "D:/DATA/2015/Sep2015/sep22/1705_10111_36MLiClpH8_3uLlane1dsDNA_150mV/events/event_00300.csv", path "D:/DATA/2015/Sep2015/sep22/1705_10111_36MLiClpH8_3uLlane1dsDNA_150mV/events/event_00301.csv", path "D:/DATA/2015/Sep2015/sep22/1705_10111_36MLiClpH8_3uLlane1dsDNA_150mV/events/event_00303.csv", path "D:/DATA/2015/Sep2015/sep22/1705_10111_36MLiClpH8_3uLlane1dsDNA_150mV/events/event_00304.csv", path "D:/DATA/2015/Sep2015/sep22/1705_10111_36MLiClpH8_3uLlane1dsDNA_150mV/events/event_00305.csv", path "D:/DATA/2015/Sep2015/sep22/1705_10111_36MLiClpH8_3uLlane1dsDNA_150mV/events/event_00306.csv", path "D:/DATA/2015/Sep2015/sep22/1705_10111_36MLiClpH8_3uLlane1dsDNA_150mV/events/event_00307.csv", path "D:/DATA/2015/Sep2015/sep22/1705_10111_36MLiClpH8_3uLlane1dsDNA_150mV/events/event_00308.csv", path "D:/DATA/2015/Sep2015/sep22/1705_10111_36MLiClpH8_3uLlane1dsDNA_150mV/events/event_00309.csv", path "D:/DATA/2015/Sep2015/sep22/1705_10111_36MLiClpH8_3uLlane1dsDNA_150mV/events/event_00310.csv", path "D:/DATA/2015/Sep2015/sep22/1705_10111_36MLiClpH8_3uLlane1dsDNA_150mV/events/event_00311.csv", path "D:/DATA/2015/Sep2015/sep22/1705_10111_36MLiClpH8_3uLlane1dsDNA_150mV/events/event_00312.csv", path "D:/DATA/2015/Sep2015/sep22/1705_10111_36MLiClpH8_3uLlane1dsDNA_150mV/events/event_00313.csv", path "D:/DATA/2015/Sep2015/sep22/1705_10111_36MLiClpH8_3uLlane1dsDNA_150mV/events/event_00314.csv", path "D:/DATA/2015/Sep2015/sep22/1705_10111_36MLiClpH8_3uLlane1dsDNA_150mV/events/event_00316.csv", path "D:/DATA/2015/Sep2015/sep22/1705_10111_36MLiClpH8_3uLlane1dsDNA_150mV/events/event_00318.csv", path "D:/DATA/2015/Sep2015/sep22/1705_10111_36MLiClpH8_3uLlane1dsDNA_150mV/events/event_00319.csv", path "D:/DATA/2015/Sep2015/sep22/1705_10111_36MLiClpH8_3uLlane1dsDNA_150mV/events/event_00321.csv", path "D:/DATA/2015/Sep2015/sep22/1705_10111_36MLiClpH8_3uLlane1dsDNA_150mV/events/event_00322.csv", path "D:/DATA/2015/Sep2015/sep22/1705_10111_36MLiClpH8_3uLlane1dsDNA_150mV/events/event_00323.csv", path "D:/DATA/2015/Sep2015/sep22/1705_10111_36MLiClpH8_3uLlane1dsDNA_150mV/events/event_00324.csv", path "D:/DATA/2015/Sep2015/sep22/1705_10111_36MLiClpH8_3uLlane1dsDNA_150mV/events/event_00326.csv", path "D:/DATA/2015/Sep2015/sep22/1705_10111_36MLiClpH8_3uLlane1dsDNA_150mV/events/event_00327.csv", path "D:/DATA/2015/Sep2015/sep22/1705_10111_36MLiClpH8_3uLlane1dsDNA_150mV/events/event_00328.csv", path "D:/DATA/2015/Sep2015/sep22/1705_10111_36MLiClpH8_3uLlane1dsDNA_150mV/events/event_00329.csv", path "D:/DATA/2015/Sep2015/sep22/1705_10111_36MLiClpH8_3uLlane1dsDNA_150mV/events/event_00330.csv", path "D:/DATA/2015/Sep2015/sep22/1705_10111_36MLiClpH8_3uLlane1dsDNA_150mV/events/event_00332.csv", path "D:/DATA/2015/Sep2015/sep22/1705_10111_36MLiClpH8_3uLlane1dsDNA_150mV/events/event_00333.csv", path "D:/DATA/2015/Sep2015/sep22/1705_10111_36MLiClpH8_3uLlane1dsDNA_150mV/events/event_00335.csv", path "D:/DATA/2015/Sep2015/sep22/1705_10111_36MLiClpH8_3uLlane1dsDNA_150mV/events/event_00336.csv", path "D:/DATA/2015/Sep2015/sep22/1705_10111_36MLiClpH8_3uLlane1dsDNA_150mV/events/event_00340.csv", path "D:/DATA/2015/Sep2015/sep22/1705_10111_36MLiClpH8_3uLlane1dsDNA_150mV/events/event_00342.csv", path "D:/DATA/2015/Sep2015/sep22/1705_10111_36MLiClpH8_3uLlane1dsDNA_150mV/events/event_00344.csv", path "D:/DATA/2015/Sep2015/sep22/1705_10111_36MLiClpH8_3uLlane1dsDNA_150mV/events/event_00345.csv", path "D:/DATA/2015/Sep2015/sep22/1705_10111_36MLiClpH8_3uLlane1dsDNA_150mV/events/event_00346.csv", path "D:/DATA/2015/Sep2015/sep22/1705_10111_36MLiClpH8_3uLlane1dsDNA_150mV/events/event_00348.csv", path "D:/DATA/2015/Sep2015/sep22/1705_10111_36MLiClpH8_3uLlane1dsDNA_150mV/events/event_00349.csv", path "D:/DATA/2015/Sep2015/sep22/1705_10111_36MLiClpH8_3uLlane1dsDNA_150mV/events/event_00351.csv", path "D:/DATA/2015/Sep2015/sep22/1705_10111_36MLiClpH8_3uLlane1dsDNA_150mV/events/event_00352.csv", path "D:/DATA/2015/Sep2015/sep22/1705_10111_36MLiClpH8_3uLlane1dsDNA_150mV/events/event_00353.csv", path "D:/DATA/2015/Sep2015/sep22/1705_10111_36MLiClpH8_3uLlane1dsDNA_150mV/events/event_00354.csv", path "D:/DATA/2015/Sep2015/sep22/1705_10111_36MLiClpH8_3uLlane1dsDNA_150mV/events/event_00355.csv", path "D:/DATA/2015/Sep2015/sep22/1705_10111_36MLiClpH8_3uLlane1dsDNA_150mV/events/event_00356.csv", path "D:/DATA/2015/Sep2015/sep22/1705_10111_36MLiClpH8_3uLlane1dsDNA_150mV/events/event_00357.csv", path "D:/DATA/2015/Sep2015/sep22/1705_10111_36MLiClpH8_3uLlane1dsDNA_150mV/events/event_00358.csv", path "D:/DATA/2015/Sep2015/sep22/1705_10111_36MLiClpH8_3uLlane1dsDNA_150mV/events/event_00359.csv", path "D:/DATA/2015/Sep2015/sep22/1705_10111_36MLiClpH8_3uLlane1dsDNA_150mV/events/event_00360.csv", path "D:/DATA/2015/Sep2015/sep22/1705_10111_36MLiClpH8_3uLlane1dsDNA_150mV/events/event_00362.csv", path "D:/DATA/2015/Sep2015/sep22/1705_10111_36MLiClpH8_3uLlane1dsDNA_150mV/events/event_00363.csv", path "D:/DATA/2015/Sep2015/sep22/1705_10111_36MLiClpH8_3uLlane1dsDNA_150mV/events/event_00364.csv", path "D:/DATA/2015/Sep2015/sep22/1705_10111_36MLiClpH8_3uLlane1dsDNA_150mV/events/event_00365.csv", path "D:/DATA/2015/Sep2015/sep22/1705_10111_36MLiClpH8_3uLlane1dsDNA_150mV/events/event_00366.csv", path "D:/DATA/2015/Sep2015/sep22/1705_10111_36MLiClpH8_3uLlane1dsDNA_150mV/events/event_00368.csv", path "D:/DATA/2015/Sep2015/sep22/1705_10111_36MLiClpH8_3uLlane1dsDNA_150mV/events/event_00369.csv", path "D:/DATA/2015/Sep2015/sep22/1705_10111_36MLiClpH8_3uLlane1dsDNA_150mV/events/event_00370.csv", path "D:/DATA/2015/Sep2015/sep22/1705_10111_36MLiClpH8_3uLlane1dsDNA_150mV/events/event_00371.csv", path "D:/DATA/2015/Sep2015/sep22/1705_10111_36MLiClpH8_3uLlane1dsDNA_150mV/events/event_00372.csv", path "D:/DATA/2015/Sep2015/sep22/1705_10111_36MLiClpH8_3uLlane1dsDNA_150mV/events/event_00373.csv", path "D:/DATA/2015/Sep2015/sep22/1705_10111_36MLiClpH8_3uLlane1dsDNA_150mV/events/event_00374.csv", path "D:/DATA/2015/Sep2015/sep22/1705_10111_36MLiClpH8_3uLlane1dsDNA_150mV/events/event_00378.csv", path "D:/DATA/2015/Sep2015/sep22/1705_10111_36MLiClpH8_3uLlane1dsDNA_150mV/events/event_00379.csv", path "D:/DATA/2015/Sep2015/sep22/1705_10111_36MLiClpH8_3uLlane1dsDNA_150mV/events/event_00380.csv", path "D:/DATA/2015/Sep2015/sep22/1705_10111_36MLiClpH8_3uLlane1dsDNA_150mV/events/event_00382.csv", path "D:/DATA/2015/Sep2015/sep22/1705_10111_36MLiClpH8_3uLlane1dsDNA_150mV/events/event_00383.csv", path "D:/DATA/2015/Sep2015/sep22/1705_10111_36MLiClpH8_3uLlane1dsDNA_150mV/events/event_00384.csv", path "D:/DATA/2015/Sep2015/sep22/1705_10111_36MLiClpH8_3uLlane1dsDNA_150mV/events/event_00385.csv", path "D:/DATA/2015/Sep2015/sep22/1705_10111_36MLiClpH8_3uLlane1dsDNA_150mV/events/event_00386.csv", path "D:/DATA/2015/Sep2015/sep22/1705_10111_36MLiClpH8_3uLlane1dsDNA_150mV/events/event_00387.csv", path "D:/DATA/2015/Sep2015/sep22/1705_10111_36MLiClpH8_3uLlane1dsDNA_150mV/events/event_00388.csv", path "D:/DATA/2015/Sep2015/sep22/1705_10111_36MLiClpH8_3uLlane1dsDNA_150mV/events/event_00389.csv", path "D:/DATA/2015/Sep2015/sep22/1705_10111_36MLiClpH8_3uLlane1dsDNA_150mV/events/event_00390.csv", path "D:/DATA/2015/Sep2015/sep22/1705_10111_36MLiClpH8_3uLlane1dsDNA_150mV/events/event_00392.csv", path "D:/DATA/2015/Sep2015/sep22/1705_10111_36MLiClpH8_3uLlane1dsDNA_150mV/events/event_00393.csv", path "D:/DATA/2015/Sep2015/sep22/1705_10111_36MLiClpH8_3uLlane1dsDNA_150mV/events/event_00395.csv", path "D:/DATA/2015/Sep2015/sep22/1705_10111_36MLiClpH8_3uLlane1dsDNA_150mV/events/event_00397.csv", path "D:/DATA/2015/Sep2015/sep22/1705_10111_36MLiClpH8_3uLlane1dsDNA_150mV/events/event_00398.csv", path "D:/DATA/2015/Sep2015/sep22/1705_10111_36MLiClpH8_3uLlane1dsDNA_150mV/events/event_00399.csv", path "D:/DATA/2015/Sep2015/sep22/1705_10111_36MLiClpH8_3uLlane1dsDNA_150mV/events/event_00400.csv", path "D:/DATA/2015/Sep2015/sep22/1705_10111_36MLiClpH8_3uLlane1dsDNA_150mV/events/event_00401.csv", path "D:/DATA/2015/Sep2015/sep22/1705_10111_36MLiClpH8_3uLlane1dsDNA_150mV/events/event_00402.csv", path "D:/DATA/2015/Sep2015/sep22/1705_10111_36MLiClpH8_3uLlane1dsDNA_150mV/events/event_00404.csv", path "D:/DATA/2015/Sep2015/sep22/1705_10111_36MLiClpH8_3uLlane1dsDNA_150mV/events/event_00405.csv", path "D:/DATA/2015/Sep2015/sep22/1705_10111_36MLiClpH8_3uLlane1dsDNA_150mV/events/event_00406.csv", path "D:/DATA/2015/Sep2015/sep22/1705_10111_36MLiClpH8_3uLlane1dsDNA_150mV/events/event_00407.csv", path "D:/DATA/2015/Sep2015/sep22/1705_10111_36MLiClpH8_3uLlane1dsDNA_150mV/events/event_00410.csv", path "D:/DATA/2015/Sep2015/sep22/1705_10111_36MLiClpH8_3uLlane1dsDNA_150mV/events/event_00411.csv", path "D:/DATA/2015/Sep2015/sep22/1705_10111_36MLiClpH8_3uLlane1dsDNA_150mV/events/event_00412.csv", path "D:/DATA/2015/Sep2015/sep22/1705_10111_36MLiClpH8_3uLlane1dsDNA_150mV/events/event_00413.csv", path "D:/DATA/2015/Sep2015/sep22/1705_10111_36MLiClpH8_3uLlane1dsDNA_150mV/events/event_00415.csv", path "D:/DATA/2015/Sep2015/sep22/1705_10111_36MLiClpH8_3uLlane1dsDNA_150mV/events/event_00416.csv", path "D:/DATA/2015/Sep2015/sep22/1705_10111_36MLiClpH8_3uLlane1dsDNA_150mV/events/event_00417.csv", path "D:/DATA/2015/Sep2015/sep22/1705_10111_36MLiClpH8_3uLlane1dsDNA_150mV/events/event_00418.csv", path "D:/DATA/2015/Sep2015/sep22/1705_10111_36MLiClpH8_3uLlane1dsDNA_150mV/events/event_00419.csv", path "D:/DATA/2015/Sep2015/sep22/1705_10111_36MLiClpH8_3uLlane1dsDNA_150mV/events/event_00420.csv", path "D:/DATA/2015/Sep2015/sep22/1705_10111_36MLiClpH8_3uLlane1dsDNA_150mV/events/event_00421.csv", path "D:/DATA/2015/Sep2015/sep22/1705_10111_36MLiClpH8_3uLlane1dsDNA_150mV/events/event_00422.csv", path "D:/DATA/2015/Sep2015/sep22/1705_10111_36MLiClpH8_3uLlane1dsDNA_150mV/events/event_00423.csv", path "D:/DATA/2015/Sep2015/sep22/1705_10111_36MLiClpH8_3uLlane1dsDNA_150mV/events/event_00424.csv", path "D:/DATA/2015/Sep2015/sep22/1705_10111_36MLiClpH8_3uLlane1dsDNA_150mV/events/event_00425.csv", path "D:/DATA/2015/Sep2015/sep22/1705_10111_36MLiClpH8_3uLlane1dsDNA_150mV/events/event_00426.csv", path "D:/DATA/2015/Sep2015/sep22/1705_10111_36MLiClpH8_3uLlane1dsDNA_150mV/events/event_00427.csv", path "D:/DATA/2015/Sep2015/sep22/1705_10111_36MLiClpH8_3uLlane1dsDNA_150mV/events/event_00428.csv", path "D:/DATA/2015/Sep2015/sep22/1705_10111_36MLiClpH8_3uLlane1dsDNA_150mV/events/event_00429.csv", path "D:/DATA/2015/Sep2015/sep22/1705_10111_36MLiClpH8_3uLlane1dsDNA_150mV/events/event_00430.csv", path "D:/DATA/2015/Sep2015/sep22/1705_10111_36MLiClpH8_3uLlane1dsDNA_150mV/events/event_00431.csv", path "D:/DATA/2015/Sep2015/sep22/1705_10111_36MLiClpH8_3uLlane1dsDNA_150mV/events/event_00434.csv", path "D:/DATA/2015/Sep2015/sep22/1705_10111_36MLiClpH8_3uLlane1dsDNA_150mV/events/event_00435.csv", path "D:/DATA/2015/Sep2015/sep22/1705_10111_36MLiClpH8_3uLlane1dsDNA_150mV/events/event_00436.csv", path "D:/DATA/2015/Sep2015/sep22/1705_10111_36MLiClpH8_3uLlane1dsDNA_150mV/events/event_00437.csv", path "D:/DATA/2015/Sep2015/sep22/1705_10111_36MLiClpH8_3uLlane1dsDNA_150mV/events/event_00439.csv", path "D:/DATA/2015/Sep2015/sep22/1705_10111_36MLiClpH8_3uLlane1dsDNA_150mV/events/event_00440.csv", path "D:/DATA/2015/Sep2015/sep22/1705_10111_36MLiClpH8_3uLlane1dsDNA_150mV/events/event_00443.csv", path "D:/DATA/2015/Sep2015/sep22/1705_10111_36MLiClpH8_3uLlane1dsDNA_150mV/events/event_00444.csv", path "D:/DATA/2015/Sep2015/sep22/1705_10111_36MLiClpH8_3uLlane1dsDNA_150mV/events/event_00445.csv", path "D:/DATA/2015/Sep2015/sep22/1705_10111_36MLiClpH8_3uLlane1dsDNA_150mV/events/event_00446.csv", path "D:/DATA/2015/Sep2015/sep22/1705_10111_36MLiClpH8_3uLlane1dsDNA_150mV/events/event_00447.csv", path "D:/DATA/2015/Sep2015/sep22/1705_10111_36MLiClpH8_3uLlane1dsDNA_150mV/events/event_00448.csv", path "D:/DATA/2015/Sep2015/sep22/1705_10111_36MLiClpH8_3uLlane1dsDNA_150mV/events/event_00449.csv", path "D:/DATA/2015/Sep2015/sep22/1705_10111_36MLiClpH8_3uLlane1dsDNA_150mV/events/event_00451.csv", path "D:/DATA/2015/Sep2015/sep22/1705_10111_36MLiClpH8_3uLlane1dsDNA_150mV/events/event_00452.csv", path "D:/DATA/2015/Sep2015/sep22/1705_10111_36MLiClpH8_3uLlane1dsDNA_150mV/events/event_00453.csv", path "D:/DATA/2015/Sep2015/sep22/1705_10111_36MLiClpH8_3uLlane1dsDNA_150mV/events/event_00454.csv", path "D:/DATA/2015/Sep2015/sep22/1705_10111_36MLiClpH8_3uLlane1dsDNA_150mV/events/event_00455.csv", path "D:/DATA/2015/Sep2015/sep22/1705_10111_36MLiClpH8_3uLlane1dsDNA_150mV/events/event_00457.csv", path "D:/DATA/2015/Sep2015/sep22/1705_10111_36MLiClpH8_3uLlane1dsDNA_150mV/events/event_00458.csv", path "D:/DATA/2015/Sep2015/sep22/1705_10111_36MLiClpH8_3uLlane1dsDNA_150mV/events/event_00460.csv", path "D:/DATA/2015/Sep2015/sep22/1705_10111_36MLiClpH8_3uLlane1dsDNA_150mV/events/event_00461.csv", path "D:/DATA/2015/Sep2015/sep22/1705_10111_36MLiClpH8_3uLlane1dsDNA_150mV/events/event_00462.csv", path "D:/DATA/2015/Sep2015/sep22/1705_10111_36MLiClpH8_3uLlane1dsDNA_150mV/events/event_00463.csv", path "D:/DATA/2015/Sep2015/sep22/1705_10111_36MLiClpH8_3uLlane1dsDNA_150mV/events/event_00464.csv", path "D:/DATA/2015/Sep2015/sep22/1705_10111_36MLiClpH8_3uLlane1dsDNA_150mV/events/event_00466.csv", path "D:/DATA/2015/Sep2015/sep22/1705_10111_36MLiClpH8_3uLlane1dsDNA_150mV/events/event_00468.csv", path "D:/DATA/2015/Sep2015/sep22/1705_10111_36MLiClpH8_3uLlane1dsDNA_150mV/events/event_00469.csv", path "D:/DATA/2015/Sep2015/sep22/1705_10111_36MLiClpH8_3uLlane1dsDNA_150mV/events/event_00470.csv", path "D:/DATA/2015/Sep2015/sep22/1705_10111_36MLiClpH8_3uLlane1dsDNA_150mV/events/event_00471.csv", path "D:/DATA/2015/Sep2015/sep22/1705_10111_36MLiClpH8_3uLlane1dsDNA_150mV/events/event_00472.csv", path "D:/DATA/2015/Sep2015/sep22/1705_10111_36MLiClpH8_3uLlane1dsDNA_150mV/events/event_00473.csv", path "D:/DATA/2015/Sep2015/sep22/1705_10111_36MLiClpH8_3uLlane1dsDNA_150mV/events/event_00475.csv", path "D:/DATA/2015/Sep2015/sep22/1705_10111_36MLiClpH8_3uLlane1dsDNA_150mV/events/event_00476.csv", path "D:/DATA/2015/Sep2015/sep22/1705_10111_36MLiClpH8_3uLlane1dsDNA_150mV/events/event_00477.csv", path "D:/DATA/2015/Sep2015/sep22/1705_10111_36MLiClpH8_3uLlane1dsDNA_150mV/events/event_00479.csv", path "D:/DATA/2015/Sep2015/sep22/1705_10111_36MLiClpH8_3uLlane1dsDNA_150mV/events/event_00480.csv", path "D:/DATA/2015/Sep2015/sep22/1705_10111_36MLiClpH8_3uLlane1dsDNA_150mV/events/event_00482.csv", path "D:/DATA/2015/Sep2015/sep22/1705_10111_36MLiClpH8_3uLlane1dsDNA_150mV/events/event_00484.csv", path "D:/DATA/2015/Sep2015/sep22/1705_10111_36MLiClpH8_3uLlane1dsDNA_150mV/events/event_00485.csv", path "D:/DATA/2015/Sep2015/sep22/1705_10111_36MLiClpH8_3uLlane1dsDNA_150mV/events/event_00486.csv", path "D:/DATA/2015/Sep2015/sep22/1705_10111_36MLiClpH8_3uLlane1dsDNA_150mV/events/event_00487.csv", path "D:/DATA/2015/Sep2015/sep22/1705_10111_36MLiClpH8_3uLlane1dsDNA_150mV/events/event_00489.csv", path "D:/DATA/2015/Sep2015/sep22/1705_10111_36MLiClpH8_3uLlane1dsDNA_150mV/events/event_00490.csv", path "D:/DATA/2015/Sep2015/sep22/1705_10111_36MLiClpH8_3uLlane1dsDNA_150mV/events/event_00491.csv", path "D:/DATA/2015/Sep2015/sep22/1705_10111_36MLiClpH8_3uLlane1dsDNA_150mV/events/event_00492.csv", path "D:/DATA/2015/Sep2015/sep22/1705_10111_36MLiClpH8_3uLlane1dsDNA_150mV/events/event_00493.csv", path "D:/DATA/2015/Sep2015/sep22/1705_10111_36MLiClpH8_3uLlane1dsDNA_150mV/events/event_00494.csv", path "D:/DATA/2015/Sep2015/sep22/1705_10111_36MLiClpH8_3uLlane1dsDNA_150mV/events/event_00495.csv", path "D:/DATA/2015/Sep2015/sep22/1705_10111_36MLiClpH8_3uLlane1dsDNA_150mV/events/event_00498.csv", path "D:/DATA/2015/Sep2015/sep22/1705_10111_36MLiClpH8_3uLlane1dsDNA_150mV/events/event_00500.csv", path "D:/DATA/2015/Sep2015/sep22/1705_10111_36MLiClpH8_3uLlane1dsDNA_150mV/events/event_00501.csv", path "D:/DATA/2015/Sep2015/sep22/1705_10111_36MLiClpH8_3uLlane1dsDNA_150mV/events/event_00502.csv", path "D:/DATA/2015/Sep2015/sep22/1705_10111_36MLiClpH8_3uLlane1dsDNA_150mV/events/event_00503.csv", path "D:/DATA/2015/Sep2015/sep22/1705_10111_36MLiClpH8_3uLlane1dsDNA_150mV/events/event_00505.csv", path "D:/DATA/2015/Sep2015/sep22/1705_10111_36MLiClpH8_3uLlane1dsDNA_150mV/events/event_00506.csv", path "D:/DATA/2015/Sep2015/sep22/1705_10111_36MLiClpH8_3uLlane1dsDNA_150mV/events/event_00507.csv", path "D:/DATA/2015/Sep2015/sep22/1705_10111_36MLiClpH8_3uLlane1dsDNA_150mV/events/event_00508.csv", path "D:/DATA/2015/Sep2015/sep22/1705_10111_36MLiClpH8_3uLlane1dsDNA_150mV/events/event_00509.csv", path "D:/DATA/2015/Sep2015/sep22/1705_10111_36MLiClpH8_3uLlane1dsDNA_150mV/events/event_00510.csv", path "D:/DATA/2015/Sep2015/sep22/1705_10111_36MLiClpH8_3uLlane1dsDNA_150mV/events/event_00511.csv", path "D:/DATA/2015/Sep2015/sep22/1705_10111_36MLiClpH8_3uLlane1dsDNA_150mV/events/event_00512.csv", path "D:/DATA/2015/Sep2015/sep22/1705_10111_36MLiClpH8_3uLlane1dsDNA_150mV/events/event_00514.csv", path "D:/DATA/2015/Sep2015/sep22/1705_10111_36MLiClpH8_3uLlane1dsDNA_150mV/events/event_00515.csv", path "D:/DATA/2015/Sep2015/sep22/1705_10111_36MLiClpH8_3uLlane1dsDNA_150mV/events/event_00516.csv", path "D:/DATA/2015/Sep2015/sep22/1705_10111_36MLiClpH8_3uLlane1dsDNA_150mV/events/event_00518.csv", path "D:/DATA/2015/Sep2015/sep22/1705_10111_36MLiClpH8_3uLlane1dsDNA_150mV/events/event_00519.csv", path "D:/DATA/2015/Sep2015/sep22/1705_10111_36MLiClpH8_3uLlane1dsDNA_150mV/events/event_00520.csv", path "D:/DATA/2015/Sep2015/sep22/1705_10111_36MLiClpH8_3uLlane1dsDNA_150mV/events/event_00521.csv", path "D:/DATA/2015/Sep2015/sep22/1705_10111_36MLiClpH8_3uLlane1dsDNA_150mV/events/event_00522.csv", path "D:/DATA/2015/Sep2015/sep22/1705_10111_36MLiClpH8_3uLlane1dsDNA_150mV/events/event_00523.csv", path "D:/DATA/2015/Sep2015/sep22/1705_10111_36MLiClpH8_3uLlane1dsDNA_150mV/events/event_00524.csv", path "D:/DATA/2015/Sep2015/sep22/1705_10111_36MLiClpH8_3uLlane1dsDNA_150mV/events/event_00525.csv", path "D:/DATA/2015/Sep2015/sep22/1705_10111_36MLiClpH8_3uLlane1dsDNA_150mV/events/event_00526.csv", path "D:/DATA/2015/Sep2015/sep22/1705_10111_36MLiClpH8_3uLlane1dsDNA_150mV/events/event_00527.csv", path "D:/DATA/2015/Sep2015/sep22/1705_10111_36MLiClpH8_3uLlane1dsDNA_150mV/events/event_00528.csv", path "D:/DATA/2015/Sep2015/sep22/1705_10111_36MLiClpH8_3uLlane1dsDNA_150mV/events/event_00529.csv", path "D:/DATA/2015/Sep2015/sep22/1705_10111_36MLiClpH8_3uLlane1dsDNA_150mV/events/event_00531.csv", path "D:/DATA/2015/Sep2015/sep22/1705_10111_36MLiClpH8_3uLlane1dsDNA_150mV/events/event_00532.csv", path "D:/DATA/2015/Sep2015/sep22/1705_10111_36MLiClpH8_3uLlane1dsDNA_150mV/events/event_00534.csv"]
  out "Total # of events":i32=405
  in  "CUSUM event summary file":path=path "D:/DATA/2015/Sep2015/sep22/1705_10111_36MLiClpH8_3uLlane1dsDNA_150mV/events_maxblockremoved.csv"
  # "'Page up/down' to \nscan through events"
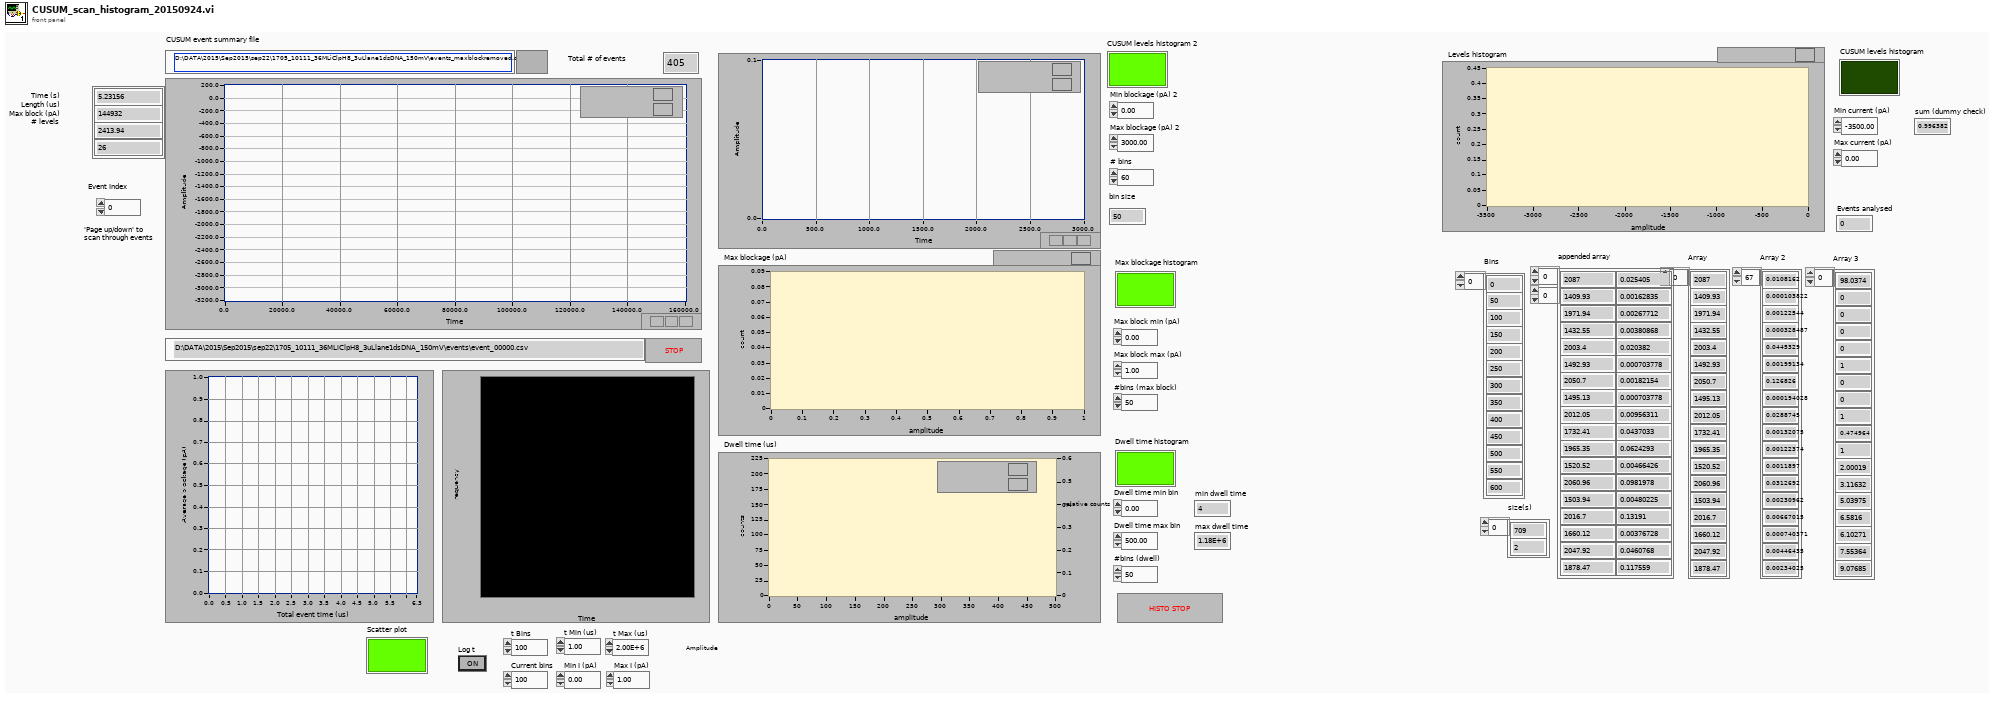
[diagram p1: front panel]
types:
  T1 = cluster{"X Values":dbl[], "Histogram: h(x)":dbl[]}
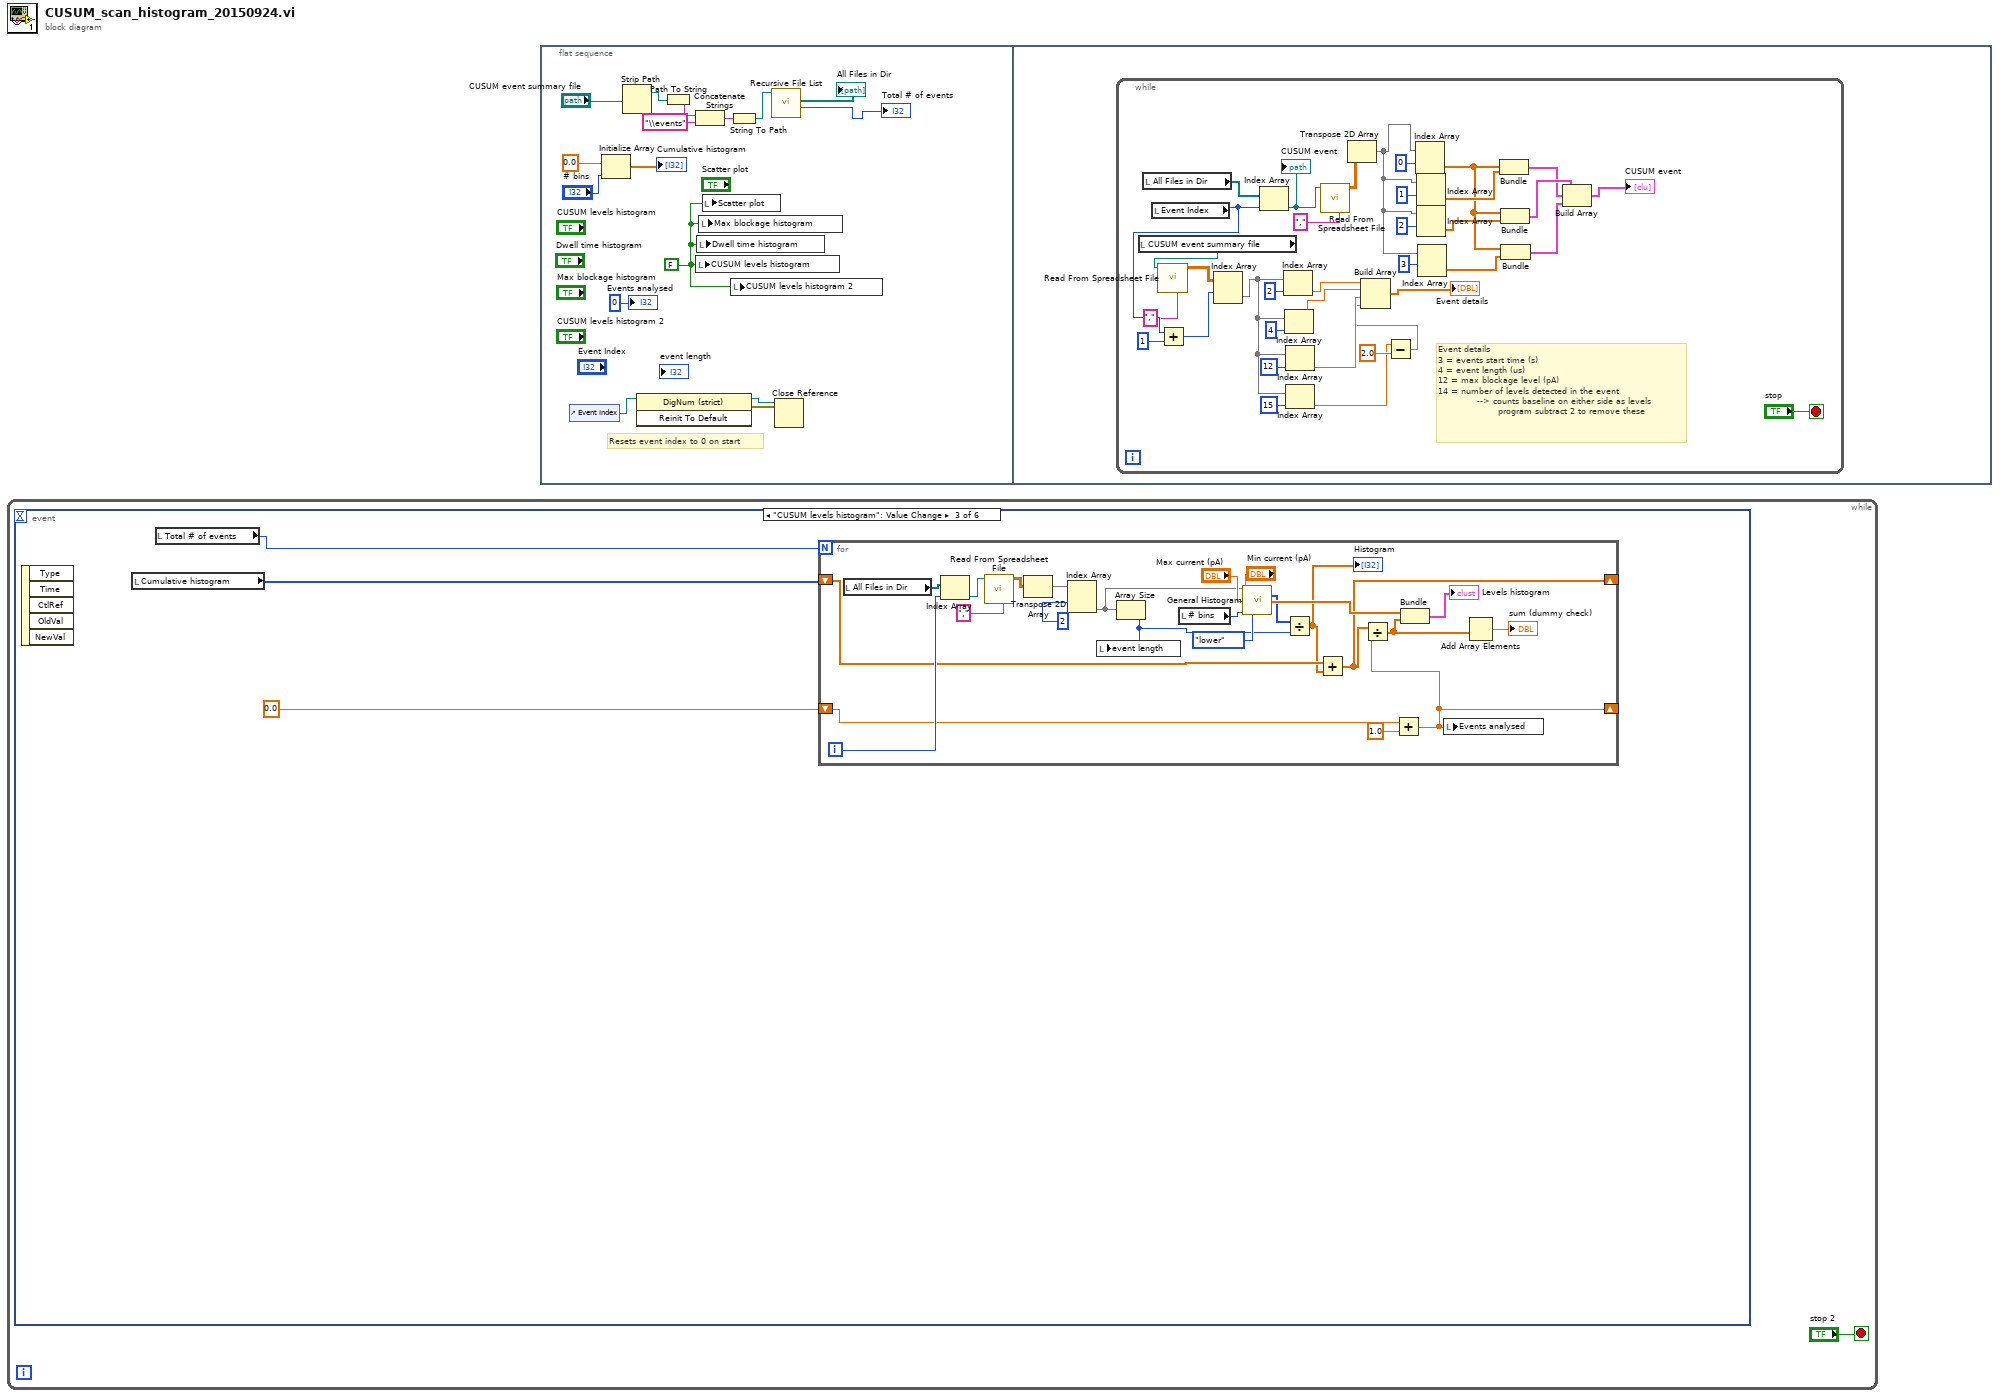
[diagram p0: block diagram]
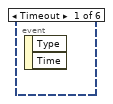
[diagram p2: hidden frame]
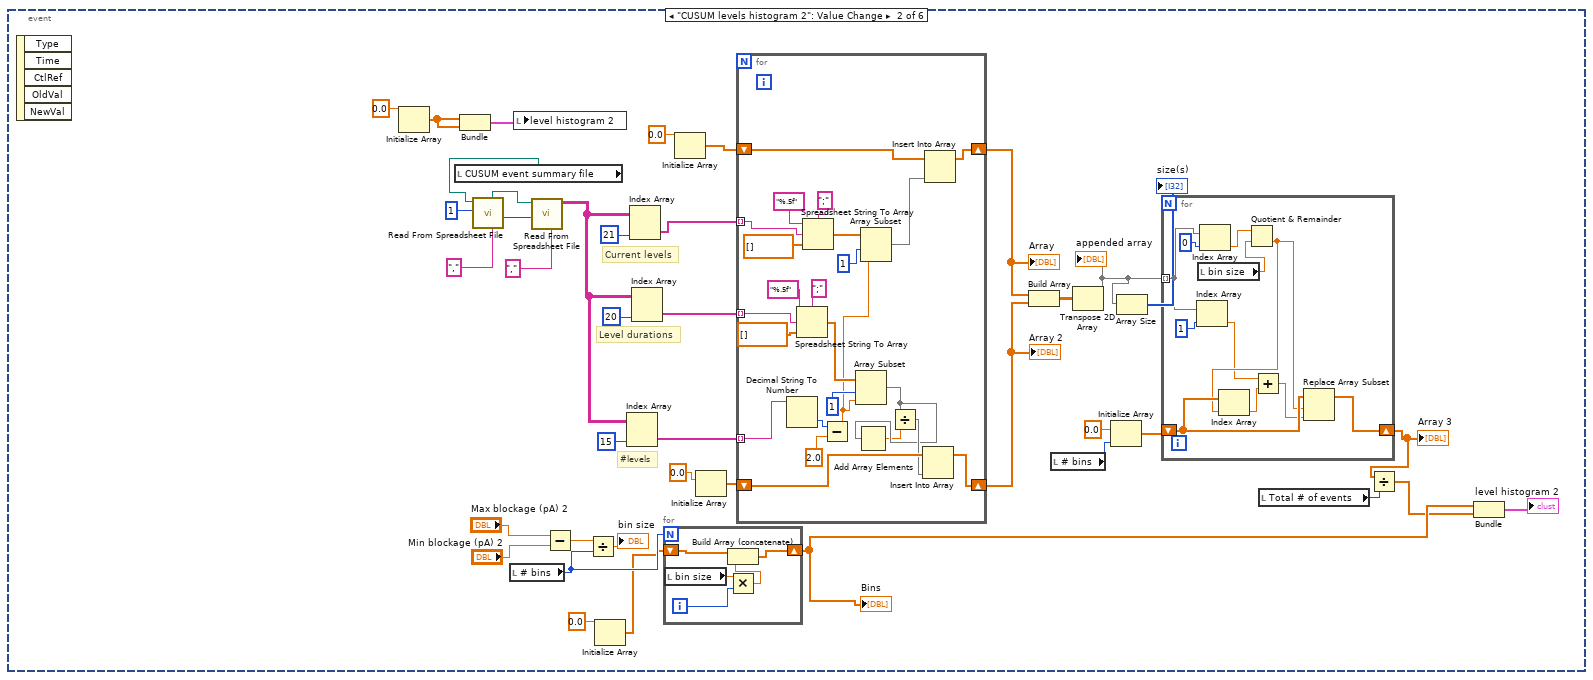
[diagram p3: hidden frame]
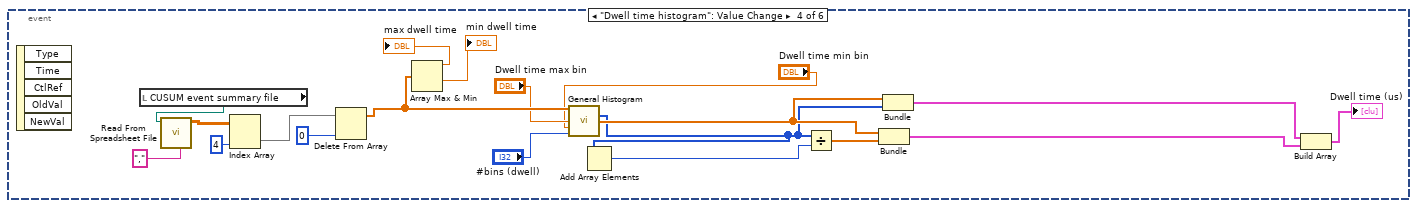
[diagram p4: hidden frame]
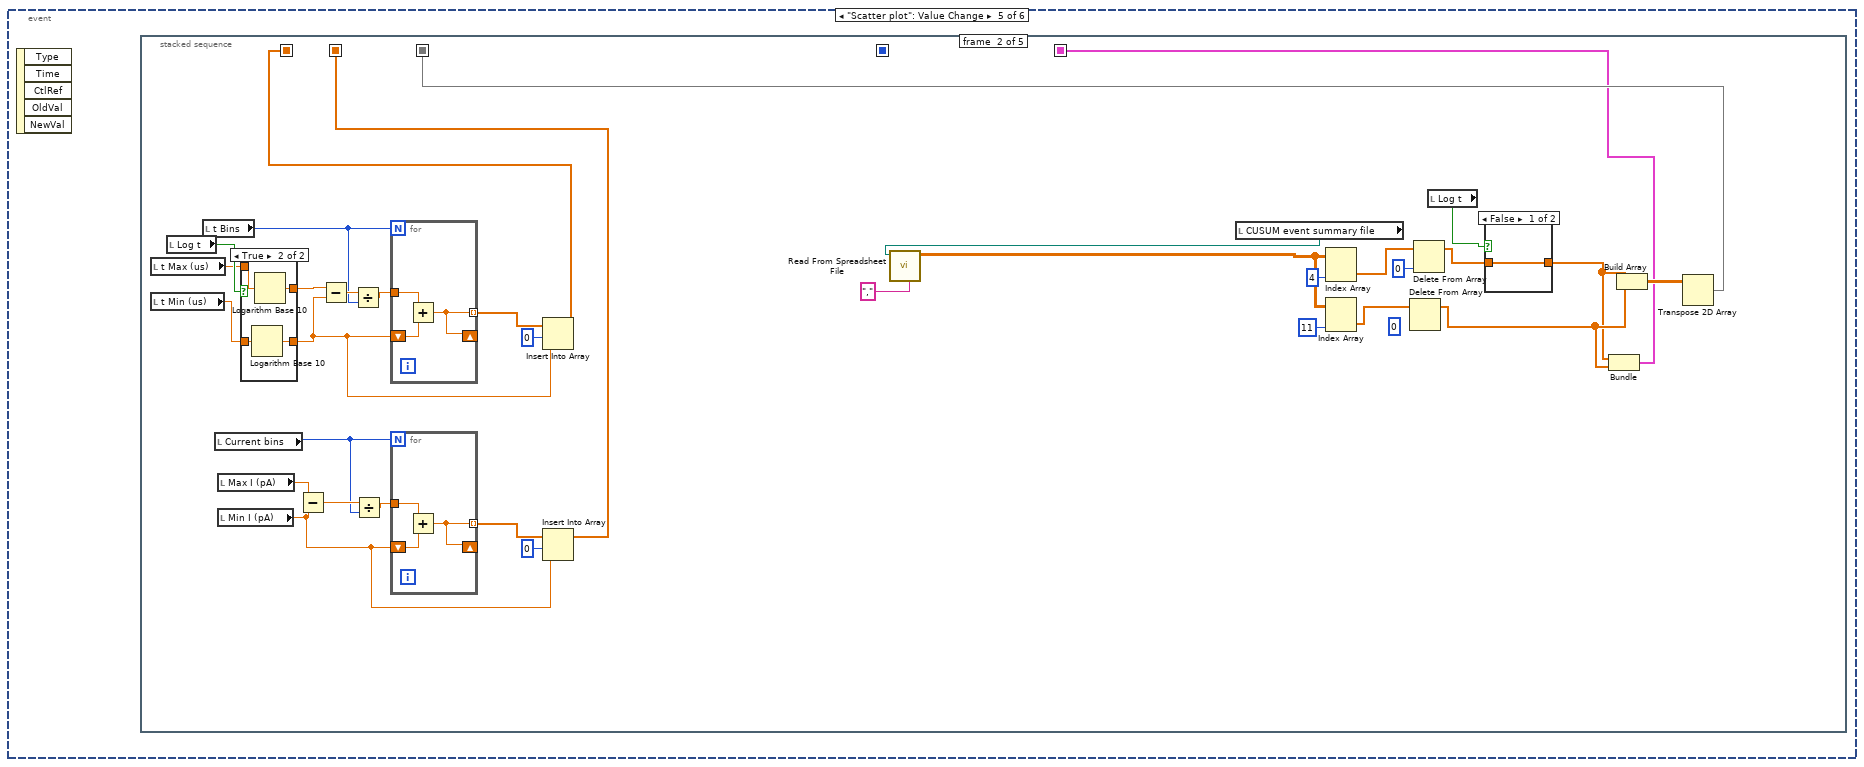
[diagram p5: hidden frame]
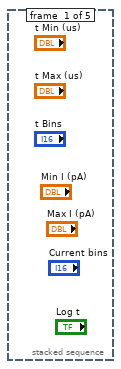
[diagram p6: hidden frame]
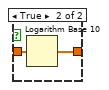
[diagram p7: hidden frame]
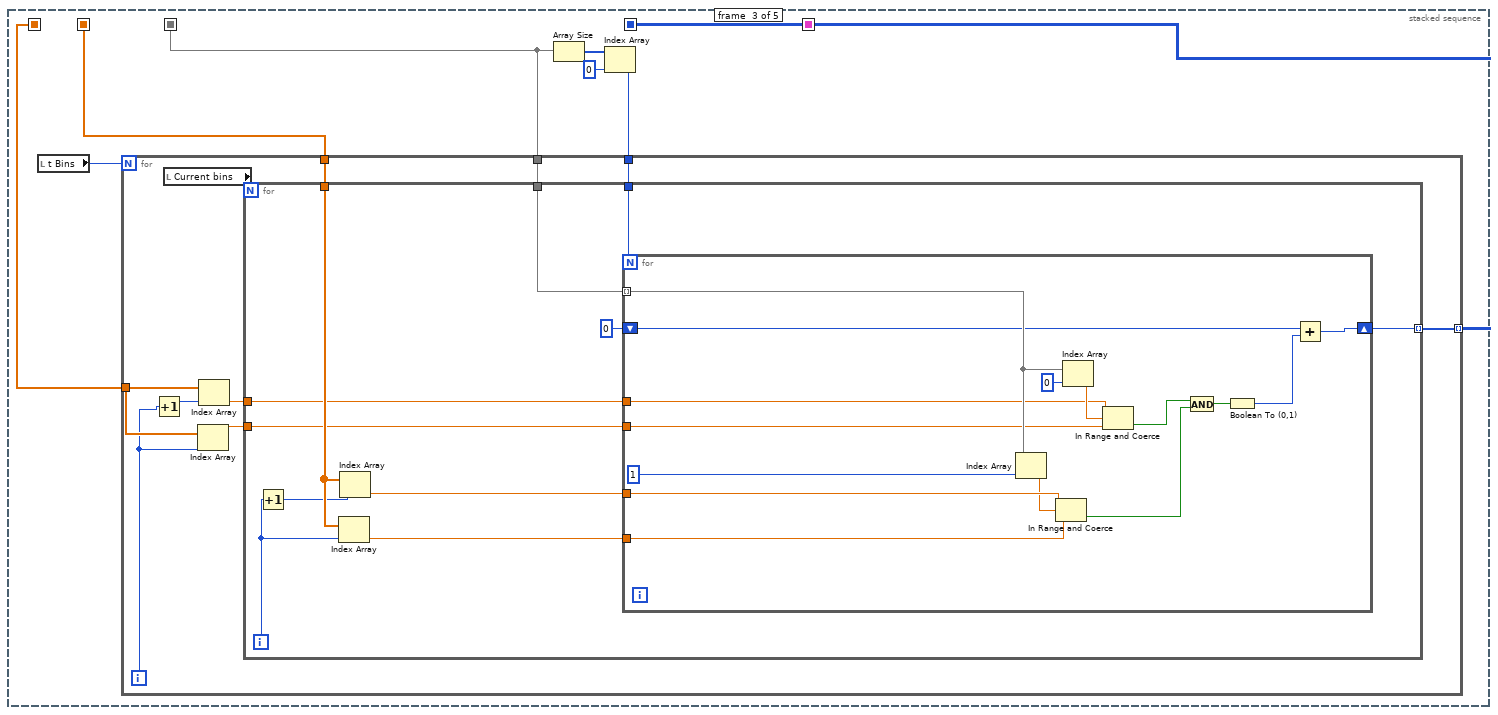
[diagram p9: hidden frame]
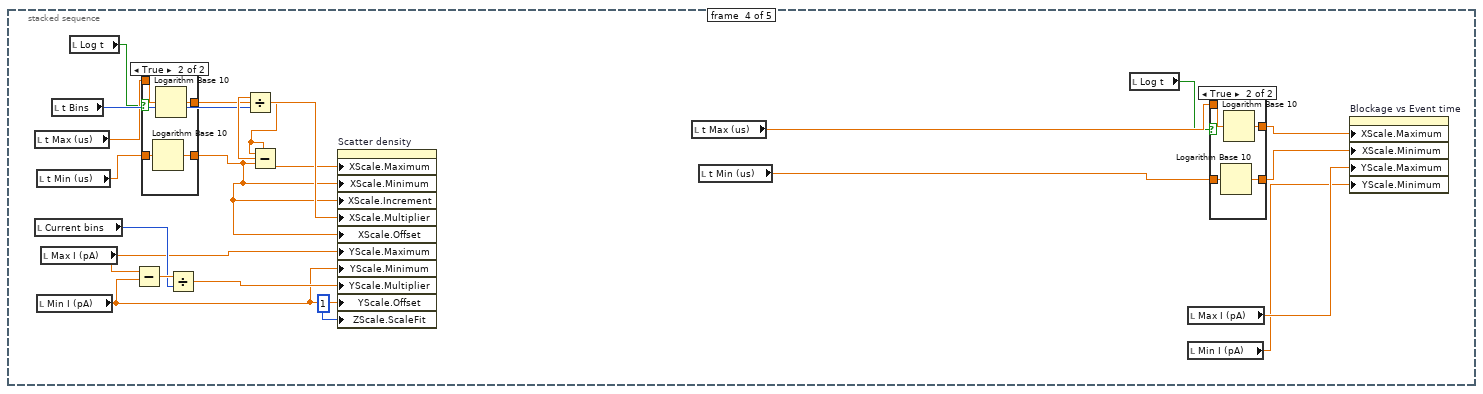
[diagram p10: hidden frame]
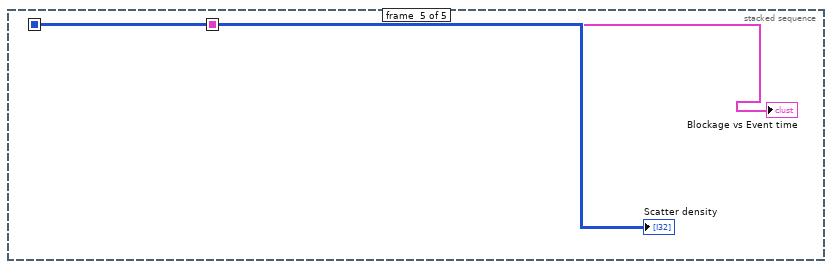
[diagram p13: hidden frame]
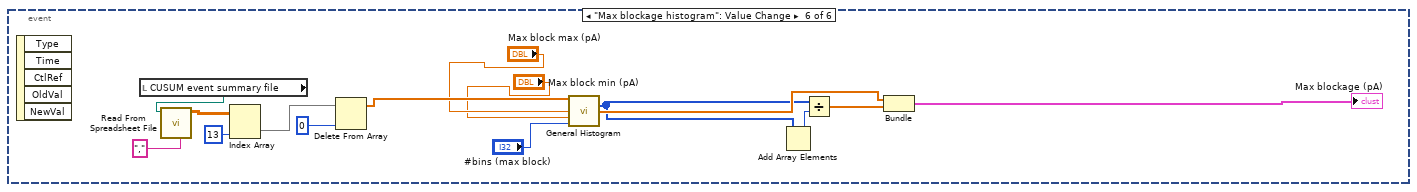
[diagram p14: hidden frame]
diagram:
  n1 = while {
    stop <- "stop 2" stop-if-true
    n2 = event shown="[2] \"CUSUM levels histogram\": Value Change" {
      selector: _ -> [_ _ _ _ _ _]
      dyn-events: _ -> [_ _ _ _ _ _]
      timeout: _ -> [_ _ _ _ _ _]
      event Timeout {
        n3 = event-data() -> ()  [unwired: 1 in, 2 out]
      }
      event "CUSUM levels histogram 2": Value Change {
        # "#levels"
        # "Level durations"
        # "Current levels"
        n4 = event-data() -> ()  [unwired: 1 in, 5 out]
        n5 = Initialize Array(0.0 ("element")) -> (w7:dbl[])  [unwired: 1 in]
        n6 = local read "CUSUM event summary file"() -> (w35:path)
        n7 = Bundle(w7, w7) -> (w8:cluster{dbl[], dbl[]})  [unwired: 1 in]
        n8 = call-poly <vilib>:"Read From Spreadsheet File.vi"("delimiter (\\t)"="," ("delimiter (\\t)"), "number of rows (all:-1)"=1 ("start of read offset (chars.:0)"), "file path (dialog if empty)"=w35) -> ("mark after read (chars.)"=w32:i32, "new file path (Not A Path if cancelled)"=w33:path)  [unwired: 4 in, 3 out]
        n9 = local read "# bins"() -> (w28:i32)
        n10 = local write "level histogram 2"(w8) -> ()
        n11 = call-poly <vilib>:"Read From Spreadsheet File.vi"("delimiter (\\t)"="," ("delimiter (\\t)"), "start of read offset (chars.:0)"=w32, "file path (dialog if empty)"=w33) -> ("all rows"=w25:string[][])  [unwired: 4 in, 4 out]
        n12 = Subtract(x="Max blockage (pA) 2", y="Min blockage (pA) 2") -> (x-y=w29:dbl)
        n13 = Divide(x=w29, y=w28) -> (x/y=→"bin size":dbl)
        n14 = Initialize Array(0.0 ("element")) -> (w11:dbl[])  [unwired: 1 in]
        n15 = Index Array(array=w25, index (col)=15 ("disabled index (col)")) -> (element=w24:string[])  [unwired: 1 in]
        n16 = Index Array(array=w25, index (col)=21 ("disabled index (col)")) -> (element=w40:string[])  [unwired: 1 in]
        n17 = Index Array(array=w25, index (col)=20 ("disabled index (col)")) -> (element=w37:string[])  [unwired: 1 in]
        n18 = for {
          N: w28 -> [_]
          shift-right: [w57] -> w10
          shift-left: w11 -> [w56]
          i -> [w54]
          n19 = local read "bin size"() -> (w55:dbl)
          n20 = Multiply(x=w55, y=w54) -> (x*y=w53:dbl)
          n21 = Build Array (concatenate)(w56, w53) -> (w57:dbl[])
        }
        "Bins" <- w10
        n22 = Initialize Array(0.0 ("element")) -> (w22:dbl[])  [unwired: 1 in]
        n23 = Initialize Array(0.0 ("element")) -> (w20:dbl[])  [unwired: 1 in]
        n24 = for {
          tunnel: w40 -> [w67] mode=indexing
          tunnel: w37 -> [w81] mode=indexing
          tunnel: w24 -> [w78] mode=indexing
          shift-right: [w74] -> w19
          shift-left: w22 -> [w73]
          shift-right: [w62] -> w18
          shift-left: w20 -> [w63]
          n25 = Decimal String To Number(string=w78) -> (number=w77:i32)  [unwired: 2 in, 1 out]
          n26 = Spreadsheet String To Array(delimiter (Tab)=";", format string="%.5f", spreadsheet string=w81, array type (2D Dbl)=dbl[] []) -> (array=w71:dbl[])
          n27 = Spreadsheet String To Array(delimiter (Tab)=";", format string="%.5f", spreadsheet string=w67, array type (2D Dbl)=dbl[] []) -> (array=w64:dbl[])
          n28 = Subtract(x=w77, y=2.0) -> (x-y=w65:dbl)
          n29 = Array Subset(array=w71, index=1, length=w65) -> (w59:dbl[])
          n30 = Add Array Elements(numeric array=w59) -> (sum=w58:dbl)
          n31 = Array Subset(array=w64, index=1, length=w65) -> (w60:dbl[])
          n32 = Divide(x=w59, y=w58) -> (x/y=w61:dbl[])
          n33 = Insert Into Array(array=w63, new element=w61) -> (w62:dbl[])  [unwired: 1 in]
          n34 = Insert Into Array(array=w73, new element=w60) -> (w74:dbl[])  [unwired: 1 in]
        }
        "Array" <- w19
        "Array 2" <- w18
        n35 = Build Array(w19, w18) -> (w17:dbl[][])
        n36 = local read "# bins"() -> (w14:i32)
        n37 = Transpose 2D Array(2D array=w17) -> (transposed array=w6:dbl[][])
        "appended array" <- w6
        n38 = Initialize Array(0.0 ("element"), w14) -> (w15:dbl[])
        n39 = Array Size(array=w6) -> (size(s)=→"size(s)":i32[])
        n40 = for {
          tunnel: w6 -> [w50] mode=indexing
          shift-right: [w47] -> w4
          shift-left: w15 -> [w46]
          n41 = Index Array(array=w50, index=1) -> (element=w43:dbl)
          n42 = local read "bin size"() -> (w49:dbl)
          n43 = Index Array(array=w50, index=0) -> (element=w48:dbl)
          n44 = Quotient & Remainder(x=w48, y=w49) -> (floor(x/y)=w45:dbl)  [unwired: 1 out]
          n45 = Index Array(array=w46, index=w45) -> (element=w44:dbl)
          n46 = Add(x=w43, y=w44) -> (x+y=w42:dbl)
          n47 = Replace Array Subset(array=w46, new element=w42, index=w45) -> (w47:dbl[])
        }
        "Array 3" <- w4
        n48 = local read "Total # of events"() -> (w3:i32)
        n49 = Divide(x=w4, y=w3) -> (x/y=w2:dbl[])
        n50 = Bundle(w10, w2) -> (→"level histogram 2":cluster{dbl[], dbl[]})  [unwired: 1 in]
      }
      event "CUSUM levels histogram": Value Change {
        n51 = event-data() -> ()  [unwired: 1 in, 5 out]
        n52 = local read "Cumulative histogram"() -> (w83:i32[])
        n53 = local read "Total # of events"() -> (w84:i32)
        n54 = for {
          N: w84 -> [_]
          shift-right: [w90] -> _
          shift-left: w83 -> [w93]
          shift-right: [w86] -> _
          shift-left: 0.0 -> [w88]
          i -> [w108]
          n55 = local read "All Files in Dir"() -> (w107:path[])
          n56 = Index Array(array=w107, index=w108) -> (element=w106:path)
          n57 = call-poly <vilib>:"Read From Spreadsheet File.vi"("delimiter (\\t)"="," ("delimiter (\\t)"), "file path (dialog if empty)"=w106) -> ("all rows"=w101:dbl[][])  [unwired: 5 in, 4 out]
          n58 = Transpose 2D Array(2D array=w101) -> (transposed array=w100:dbl[][])
          n59 = Index Array(array=w100, index (row)=2 ("index")) -> (element=w97:dbl[])  [unwired: 1 in]
          n60 = Array Size(array=w97) -> (size(s)=w95:i32)
          n61 = local write "event length"(w95) -> ()
          n62 = local read "# bins"() -> (w94:i32)
          n63 = call <vilib>:"General Histogram.vi"("X"=w97, "max"="Max current (pA)", "min"="Min current (pA)", "# bins"=w94, "inclusion"=enum32{"lower", "upper"}."lower") -> ("Histogram"=w96:i32[], "Axis"=w99:dbl[])  [unwired: 6 in, 3 out]
          n64 = Divide(x=w96, y=w95) -> (x/y=w91:dbl[])
          "Histogram" <- w91
          n65 = Add(x=w93, y=w91) -> (x+y=w90:dbl[])
          n66 = Add(x=w88, y=1.0) -> (x+y=w86:dbl)
          n67 = Divide(x=w90, y=w86) -> (x/y=w89:dbl[])
          n68 = Bundle("Axis"=w99, w89) -> (→"Levels histogram":cluster{"Axis":dbl[], dbl[]})  [unwired: 1 in]
          n69 = local write "Events analysed"(w86) -> ()
          n70 = Add Array Elements(numeric array=w89) -> (sum=→"sum (dummy check)":dbl)
        }
      }
      event "Dwell time histogram": Value Change {
        n71 = event-data() -> ()  [unwired: 1 in, 5 out]
        n72 = local read "CUSUM event summary file"() -> (w126:path)
        n73 = call-poly <vilib>:"Read From Spreadsheet File.vi"("delimiter (\\t)"="," ("delimiter (\\t)"), "file path (dialog if empty)"=w126) -> ("all rows"=w127:dbl[][])  [unwired: 5 in, 4 out]
        n74 = Index Array(array=w127, index (col)=4 ("disabled index (col)")) -> (element=w124:dbl[])  [unwired: 1 in]
        n75 = Delete From Array(array=w124, index=0) -> (array with subset deleted=w122:dbl[])  [unwired: 1 in, 1 out]
        n76 = Array Max & Min(array=w122) -> (max value=→"max dwell time":dbl, min value=→"min dwell time":dbl)  [unwired: 2 out]
        n77 = call <vilib>:"General Histogram.vi"("X"=w122, "max"="Dwell time max bin", "min"="Dwell time min bin", "# bins"="#bins (dwell)") -> ("Histogram"=w111:i32[], "Axis"=w114:dbl[])  [unwired: 7 in, 3 out]
        n78 = Add Array Elements(numeric array=w111) -> (sum=w110:i32)
        n79 = Divide(x=w111, y=w110) -> (x/y=w118:dbl[])
        n80 = Bundle("Axis"=w114, w118) -> (w113:cluster{"Axis":dbl[], dbl[]})  [unwired: 1 in]
        n81 = Bundle("Axis"=w114, "Histogram"=w111) -> (w112:cluster{"Axis":dbl[], "Histogram":i32[]})  [unwired: 1 in]
        n82 = Build Array(w112, w113) -> (→"Dwell time (us)":cluster{"Axis":dbl[], "Histogram":dbl[]}[])
      }
      event "Scatter plot": Value Change {
        n83 = event-data() -> ()  [unwired: 1 in, 5 out]
        n84 = stacked-sequence {
          seq-local: [_ w158 _ _ _] -> [_ _ w183 _ _]
          seq-local: [_ w152 _ _ _] -> [_ _ w178 _ _]
          seq-local: [_ w154 _ _ _] -> [_ _ w182 _ _]
          seq-local: [_ _ w177 _ _] -> [_ _ _ _ w255]
          seq-local: [_ w137 _ _ _] -> [_ _ _ _ w254]
          frame #0 {
          }
          frame #1 {
            (unwired) 0 ("index")
            n85 = local read "t Max (us)"() -> (w135:dbl)
            n86 = local read "t Min (us)"() -> (w133:dbl)
            n87 = local read "Log t"() -> (w136:bool)
            n88 = local read "t Bins"() -> (w150:i16)
            n89 = local read "Current bins"() -> (w146:i16)
            n90 = local read "Max I (pA)"() -> (w161:dbl)
            n91 = local read "Min I (pA)"() -> (w155:dbl)
            n92 = case shown="True" w136 {
              tunnel: w135 -> [w166 w170]
              tunnel: [w166 w169] -> w134
              tunnel: w133 -> [w165 w168]
              tunnel: [w165 w167] -> w132
              frame False {
              }
              frame True {
                n93 = Logarithm Base 10(1:w168) -> (0:w167:dbl)
                n94 = Logarithm Base 10(1:w170) -> (0:w169:dbl)
              }
            }
            n95 = Subtract(x=w161, y=w155) -> (x-y=w148:dbl)
            n96 = Subtract(x=w134, y=w132) -> (x-y=w151:dbl)
            n97 = Divide(x=w151, y=w150) -> (x/y=w149:dbl)
            n98 = Divide(x=w148, y=w146) -> (x/y=w147:dbl)
            n99 = for {
              N: w150 -> [_]
              tunnel: w149 -> [w176]
              shift-right: [w174] -> _
              shift-left: w132 -> [w175]
              tunnel: [w174] -> w160 mode=indexing
              n100 = Add(x=w176, y=w175) -> (x+y=w174:dbl)
            }
            n101 = for {
              N: w146 -> [_]
              tunnel: w147 -> [w173]
              shift-right: [w171] -> _
              shift-left: w155 -> [w172]
              tunnel: [w171] -> w156 mode=indexing
              n102 = Add(x=w173, y=w172) -> (x+y=w171:dbl)
            }
            n103 = Insert Into Array(array=w160, index=0, new element=w132) -> (w158:dbl[])
            n104 = Insert Into Array(array=w156, index=0, new element=w155) -> (w154:dbl[])
            n105 = local read "CUSUM event summary file"() -> (w139:path)
            n106 = call-poly <vilib>:"Read From Spreadsheet File.vi"("delimiter (\\t)"="," ("delimiter (\\t)"), "file path (dialog if empty)"=w139) -> ("all rows"=w144:dbl[][])  [unwired: 5 in, 4 out]
            n107 = Index Array(array=w144, index (col)=4 ("disabled index (col)")) -> (element=w141:dbl[])  [unwired: 1 in]
            n108 = Index Array(array=w144, index (col)=11) -> (element=w145:dbl[])  [unwired: 1 in]
            n109 = Delete From Array(array=w145) -> (array with subset deleted=w138:dbl[])  [unwired: 2 in, 1 out]
            n110 = Delete From Array(array=w141, index=0) -> (array with subset deleted=w131:dbl[])  [unwired: 1 in, 1 out]
            n111 = local read "Log t"() -> (w129:bool)
            n112 = case shown="False" w129 {
              tunnel: w131 -> [w162 w164]
              tunnel: [w162 w163] -> w130
              frame False {
              }
              frame True {
                n113 = Logarithm Base 10(1:w164) -> (0:w163:dbl[])
              }
            }
            n114 = Bundle("all rows"=w130, "all rows"=w138) -> (w137:cluster{"all rows":dbl[], "all rows":dbl[]})  [unwired: 1 in]
            n115 = Build Array(w130, w138) -> (w153:dbl[][])
            n116 = Transpose 2D Array(2D array=w153) -> (transposed array=w152:dbl[][])
          }
          frame #2 {
            n117 = local read "t Bins"() -> (w184:i16)
            n118 = Array Size(array=w178) -> (size(s)=w181:i32[])
            n119 = Index Array(array=w181, index=0) -> (element=w179:i32)
            n120 = for {
              N: w184 -> [_]
              tunnel: w183 -> [w194]
              tunnel: w182 -> [w192]
              tunnel: w179 -> [w191]
              tunnel: w178 -> [w190]
              tunnel: [w187] -> w177 mode=indexing
              i -> [w185]
              n121 = Increment(x=w185) -> (x+1=w186:i32)
              n122 = local read "Current bins"() -> (w193:i16)
              n123 = Index Array(array=w194, index=w185) -> (element=w188:dbl)
              n124 = Index Array(array=w194, index=w186) -> (element=w189:dbl)
              n125 = for {
                N: w193 -> [_]
                tunnel: w192 -> [w205]
                tunnel: w191 -> [w204]
                tunnel: w190 -> [w203]
                tunnel: w189 -> [w199]
                tunnel: w188 -> [w198]
                tunnel: [w197] -> w187 mode=indexing
                i -> [w196]
                n126 = Increment(x=w196) -> (x+1=w195:i32)
                n127 = Index Array(array=w205, index=w196) -> (element=w200:dbl)
                n128 = Index Array(array=w205, index=w195) -> (element=w201:dbl)
                n129 = for {
                  N: w204 -> [_]
                  tunnel: w203 -> [w214] mode=indexing
                  shift-right: [w206] -> w197
                  shift-left: 0 -> [w207]
                  tunnel: w201 -> [w220]
                  tunnel: w200 -> [w219]
                  tunnel: w199 -> [w213]
                  tunnel: w198 -> [w212]
                  n130 = Index Array(array=w214, index=1) -> (element=w217:dbl)
                  n131 = In Range and Coerce(upper limit=w220, x=w217, lower limit=w219) -> (In Range?=w210:bool)  [unwired: 1 out]
                  n132 = Index Array(array=w214, index=0) -> (element=w216:dbl)
                  n133 = In Range and Coerce(upper limit=w213, x=w216, lower limit=w212) -> (In Range?=w211:bool)  [unwired: 1 out]
                  n134 = And(x=w211, y=w210) -> (x .and. y?=w209:bool)
                  n135 = Boolean To (0,1)(Boolean=w209) -> (0, 1=w208:i16)
                  n136 = Add(x=w207, y=w208) -> (x+y=w206:i32)
                }
              }
            }
          }
          frame #3 {
            n137 = local read "t Max (us)"() -> (w230:dbl)
            n138 = local read "Current bins"() -> (w239:i16)
            n139 = local read "t Min (us)"() -> (w229:dbl)
            n140 = local read "Min I (pA)"() -> (w233:dbl)
            n141 = local read "Max I (pA)"() -> (w234:dbl)
            n142 = local read "t Bins"() -> (w236:i16)
            n143 = local read "Log t"() -> (w226:bool)
            n144 = Subtract(x=w234, y=w233) -> (x-y=w240:dbl)
            n145 = case shown="True" w226 {
              tunnel: w230 -> [w249 w253]
              tunnel: [w249 w252] -> w227
              tunnel: w229 -> [w248 w251]
              tunnel: [w248 w250] -> w228
              frame False {
              }
              frame True {
                n146 = Logarithm Base 10(1:w251) -> (0:w250:dbl)
                n147 = Logarithm Base 10(1:w253) -> (0:w252:dbl)
              }
            }
            n148 = Divide(x=w240, y=w239) -> (x/y=w238:dbl)
            n149 = Subtract(x=w227, y=w228) -> (x-y=w237:dbl)
            n150 = Divide(x=w237, y=w236) -> (x/y=w235:dbl)
            n151 = property on="Scatter density" class="IntGraph (strict)"("XScale.Maximum"=w227, "XScale.Minimum"=w228, "XScale.Increment"=w228, "XScale.Multiplier"=w235, "XScale.Offset"=w228, "YScale.Maximum"=w234, "YScale.Minimum"=w233, "YScale.Multiplier"=w238, "YScale.Offset"=w233, "ZScale.ScaleFit"=u8 1 ("Z Scale.Scale Fit")) -> ()  [unwired: 2 in, 2 out]
            n152 = local read "t Max (us)"() -> (w225:dbl)
            n153 = local read "t Min (us)"() -> (w223:dbl)
            n154 = local read "Log t"() -> (w221:bool)
            n155 = local read "Max I (pA)"() -> (w232:dbl)
            n156 = local read "Min I (pA)"() -> (w231:dbl)
            n157 = case shown="True" w221 {
              tunnel: w225 -> [w243 w247]
              tunnel: [w243 w246] -> w224
              tunnel: w223 -> [w242 w245]
              tunnel: [w242 w244] -> w222
              frame False {
              }
              frame True {
                n158 = Logarithm Base 10(1:w245) -> (0:w244:dbl)
                n159 = Logarithm Base 10(1:w247) -> (0:w246:dbl)
              }
            }
            n160 = property on="Blockage vs Event time" class="XYGraph (strict)"("XScale.Maximum"=w224, "XScale.Minimum"=w222, "YScale.Maximum"=w232, "YScale.Minimum"=w231) -> ()  [unwired: 2 in, 2 out]
          }
          frame #4 {
            "Scatter density" <- w255
            "Blockage vs Event time" <- w254
          }
        }
      }
      event "Max blockage histogram": Value Change {
        n161 = event-data() -> ()  [unwired: 1 in, 5 out]
        n162 = local read "CUSUM event summary file"() -> (w269:path)
        n163 = call-poly <vilib>:"Read From Spreadsheet File.vi"("delimiter (\\t)"="," ("delimiter (\\t)"), "file path (dialog if empty)"=w269) -> ("all rows"=w270:dbl[][])  [unwired: 5 in, 4 out]
        n164 = Index Array(array=w270, index (col)=13 ("disabled index (col)")) -> (element=w267:dbl[])  [unwired: 1 in]
        n165 = Delete From Array(array=w267, index=0) -> (array with subset deleted=w265:dbl[])  [unwired: 1 in, 1 out]
        n166 = call <vilib>:"General Histogram.vi"("X"=w265, "max"="Max block max (pA)", "min"="Max block min (pA)", "# bins"="#bins (max block)") -> ("Histogram"=w257:i32[], "Axis"=w261:dbl[])  [unwired: 7 in, 3 out]
        n167 = Add Array Elements(numeric array=w257) -> (sum=w258:i32)
        n168 = Divide(x=w257, y=w258) -> (x/y=w262:dbl[])
        n169 = Bundle("Axis"=w261, w262) -> (→"Max blockage (pA)":cluster{"Axis":dbl[], dbl[]})  [unwired: 1 in]
      }
    }
  }
  n170 = flat-sequence {
    frame #0 {
      w271 = FALSE ("Accumulate histogram")
      # "Resets event index to 0 on start"
      n171 = control-ref of="Event Index"() -> (w285:refnum<vi>)
      n172 = Initialize Array(0.0 ("element"), "# bins") -> (→"Cumulative histogram":dbl[])
      n173 = Strip Path(path="CUSUM event summary file") -> (stripped path=w277:path)  [unwired: 1 out]
      n174 = invoke class="DigNum (strict)" method="Reinit To Default"(reference=w285) -> (reference out=w284:refnum<vi>, error out=w283:errorcluster)  [unwired: 2 in, 1 out]
      n175 = Path To String(path=w277) -> (string=w276:string)
      n176 = Concatenate Strings(w276, "\\events" ("string")) -> (w274:string)
      n177 = local write "CUSUM levels histogram"(w271) -> ()
      n178 = local write "Dwell time histogram"(w271) -> ()
      n179 = local write "Max blockage histogram"(w271) -> ()
      n180 = local write "Scatter plot"(w271) -> ()
      n181 = String To Path(string=w274) -> (path=w273:path)
      n182 = local write "CUSUM levels histogram 2"(w271) -> ()
      n183 = call <vilib>:"Recursive File List.vi"("Folder Path"=w273) -> ("Number of Files"=→"Total # of events":i32, "All Files in Dir"=→"All Files in Dir":path[])  [unwired: 6 in, 3 out]
      n184 = Close Reference(reference=w284, error in (no error)=w283) -> ()  [unwired: 1 out]
      "Events analysed" <- 0
    }
    frame #1 {
      n185 = while {
        stop <- "stop" stop-if-true
        # "Event details\n3 = events start time (s)\n4 = event length (us)\n12 = max blockage level (pA)\n14 = number of levels detected in the event\n             --> counts baseline on either side as levels\n                    program subtract 2 to remove these"
        n186 = local read "CUSUM event summary file"() -> (w311:path)
        n187 = local read "All Files in Dir"() -> (w322:path[])
        n188 = local read "Event Index"() -> (w302:i32)
        n189 = call-poly <vilib>:"Read From Spreadsheet File.vi"("delimiter (\\t)"="," ("delimiter (\\t)"), "file path (dialog if empty)"=w311) -> ("all rows"=w310:dbl[][])  [unwired: 5 in, 4 out]
        n190 = Add(x=w302, y=1) -> (x+y=w303:i32)
        n191 = Index Array(array=w310, index (row)=w303) -> (element=w300:dbl[])  [unwired: 1 in]
        n192 = Index Array(array=w322, index=w302) -> (element=w321:path)
        "CUSUM event" <- w321
        n193 = Index Array(array=w300, index=2) -> (element=w309:dbl)
        n194 = Index Array(array=w300, index=4) -> (element=w308:dbl)
        n195 = Index Array(array=w300, index=12) -> (element=w307:dbl)
        n196 = Index Array(array=w300, index=15) -> (element=w297:dbl)
        n197 = call-poly <vilib>:"Read From Spreadsheet File.vi"("delimiter (\\t)"="," ("delimiter (\\t)"), "file path (dialog if empty)"=w321) -> ("all rows"=w314:dbl[][])  [unwired: 5 in, 4 out]
        n198 = Transpose 2D Array(2D array=w314) -> (transposed array=w288:dbl[][])
        n199 = Subtract(x=w297, y=2.0) -> (x-y=w296:dbl)
        n200 = Build Array(w309, w308, w307, w296) -> (→"Event details":dbl[])
        n201 = Index Array(array=w288, index (row)=0 ("index")) -> (element=w290:dbl[])  [unwired: 1 in]
        n202 = Index Array(array=w288, index (row)=1 ("index")) -> (element=w317:dbl[])  [unwired: 1 in]
        n203 = Index Array(array=w288, index (row)=2 ("index")) -> (element=w316:dbl[])  [unwired: 1 in]
        n204 = Index Array(array=w288, index (row)=3 ("index")) -> (element=w289:dbl[])  [unwired: 1 in]
        n205 = Bundle(w290, w317) -> (w312:cluster{dbl[], dbl[]})  [unwired: 1 in]
        n206 = Bundle(w290, w316) -> (w313:cluster{dbl[], dbl[]})  [unwired: 1 in]
        n207 = Bundle(w290, w289) -> (w291:cluster{dbl[], dbl[]})  [unwired: 1 in]
        n208 = Build Array(w313, w312, w291) -> (→"CUSUM event":cluster{dbl[], dbl[]}[])
      }
    }
  }
